vi "cursor window logic V3.vi"(4 "h. offset":dbl, 6 "CursIdx":i32, 7 "cursor window action":T2=enum."check", 8 "window":dbl=nan, 9 "center":dbl=nan, 10 "cursor window in":refnum<vi>, 11 "cursor window init":T1={"left"=2378.60310421286, "right "=2421.6740576496672, "center"=2421.6740576496672, "window"=2421.6740576496672, "cursors"=[], "relative"=0, "absolute"=0, "fixed vertical offset"=2421.6740576496672, "vertical offset"=2421.6740576496672, "skew"=2421.6740576496672, "default window frac"=2421.6740576496672, "kind"=enum."skewed", "skew.left"=2421.6740576496672, "skew.right"=2421.6740576496672, "Plot ref"=refnum, "wing order"=enum."back"}) -> (2 "cursor window out":refnum<vi>, 3 "cursor window out":T1={"left"=2378.60310421286, "right "=2421.6740576496672, "center"=2421.6740576496672, "window"=2421.6740576496672, "cursors"=[], "relative"=0, "absolute"=0, "fixed vertical offset"=2421.6740576496672, "vertical offset"=2421.6740576496672, "skew"=2421.6740576496672, "default window frac"=2421.6740576496672, "kind"=enum."skewed", "skew.left"=2421.6740576496672, "skew.right"=2421.6740576496672, "Plot ref"=refnum, "wing order"=enum."back"})   [LabVIEW 2018]
uses:
  stack action -- control.ctl
  cursor window action.ctl
  cursor winow.ctl
  cursor window state.ctl
  cursor action.ctl
  cursor sate.ctl
  range multiplier action.ctl
  2Dwindow.ctl
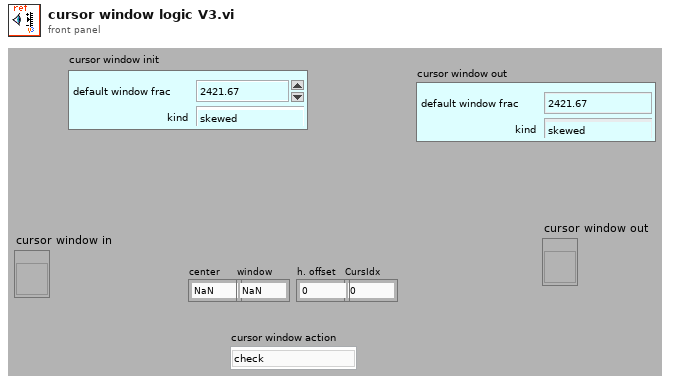
[diagram p1: front panel]
types:
  T1 = typedef "cursor winow.ctl" = cluster{"left":dbl, "right ":dbl, "center":dbl, "window":dbl, "cursors":i32[], "relative":i32, "absolute":i32, "fixed vertical offset":dbl, "vertical offset":dbl, "skew":dbl, "default window frac":dbl, "kind":enum16{"symmetric", "skewed", "fancy"}, "skew.left":dbl, "skew.right":dbl, "Plot ref":refnum<vi>, "wing order":enum16{"forw", "back"}}
  T2 = typedef "cursor window action.ctl" = enum16{"balance", "h. offset change", "cursor moves", "change center", "change window", "init", "check", "reset", "set y to middle", "idle", "-write all Y", "-write left.X", "-write center.X", "-write right.X", "-write all X", "-change center", "-change window", "-change skew", "-read cursor 2", "-read cursor 1", "-read cursor 0", "-read all cursors", "-reset", "-read plot scale", "-set y to middle", "-Q: center.Y is visible", "-Q: window is visible", "-parse center.Y", "-right left from center", "-left move", "-right move", "-set center.Y", "-empty", "-set cursors to default", "-check", "-write center.Y", "-copy cursor 1", "-copy cursor 0", "-copy cursor 2", "move right", "move left", "shrink", "broaden", "skew up", "skew down", "-write plot scale", "zoom X", "change cen&win", "zoom to all data", "color--red", "color--green", "color--yellow", "read", "zoom out", "zoom in", "slide right", "slide left", "set range aspect ratio to 1"}
  T3 = typedef "cursor window state.ctl" = cluster{"right.Y":dbl, "right.X":dbl, "left.X":dbl, "left.Y":dbl, "center.X":dbl, "center.Y":dbl, "scale.x.max":dbl, "scale.x.min":dbl, "scale.y.range":dbl, "scale.y.min":dbl, "scale.x.range":dbl, "scale.y.max":dbl, "skew":dbl, "cursor":i32, "scale.x.center":dbl, "scale.x.halfwidth":dbl, "scale.y.center":dbl, "scale.y.halfwidth":dbl}
  T4 = typedef "stack action -- control.ctl" = enum16{"push", "pop", "check", "init"}
  T5 = cluster{"center":dbl, "window":dbl, "h.offset":dbl, "cursor window":T1}
  T6 = cluster{"right.Y":dbl, "right.X":dbl, "left.X":dbl, "left.Y":dbl, "center.X":dbl, "center.Y":dbl, "scale.x.max":dbl, "scale.x.min":dbl, "scale.y.range":dbl, "scale.y.min":dbl, "scale.x.range":dbl, "scale.y.max":dbl, "skew":dbl, "cursor":i32, "scale.x.center":dbl, "scale.x.halfwidth":dbl, "scale.y.center":dbl, "scale.y.halfwidth":dbl}
  T7 = cluster{"left":dbl, "right ":dbl, "center":dbl, "window":dbl, "cursors":i32[], "relative":i32, "absolute":i32, "fixed vertical offset":dbl, "vertical offset":dbl, "skew":dbl, "default window frac":dbl, "kind":enum16{"symmetric", "skewed", "fancy"}, "skew.left":dbl, "skew.right":dbl, "Plot ref":refnum<vi>, "wing order":enum16{"forw", "back"}}
  T8 = typedef "cursor action.ctl" = enum16{"range", "read", "write", "check", "zoom out", "smart zoom out", "zoom to aspect ratio 1", "zoom to win", "zoom out 20%", "zoom in 20%", "-empty", "smart zoom out&aspect", "move range left 20%", "move range right 20%", "move range up 20%", "move range down 20%", "zoom to X win", "zoom to Y win", "zoom out X", "zoom out Y", "zoom in X", "zoom in Y", "check plot scale"}
  T9 = typedef "2Dwindow.ctl" = cluster{"window y":dbl, "center x":dbl, "center y":dbl, "window x":dbl}
  T10 = typedef "range multiplier action.ctl" = enum16{"shift", "zoom", "check"}
  T11 = typedef "comparison control.ctl" = enum16{"not a number", "above", "in range", "below"}
  T12 = typedef "2Dwindow-bounds.ctl" = cluster{"min y":dbl, "max x":dbl, "min x":dbl, "max y":dbl}
  T13 = typedef "cursor sate.ctl" = enum16{"normal", "alert", "fuzzy", "interesting", "boring", "colored"}
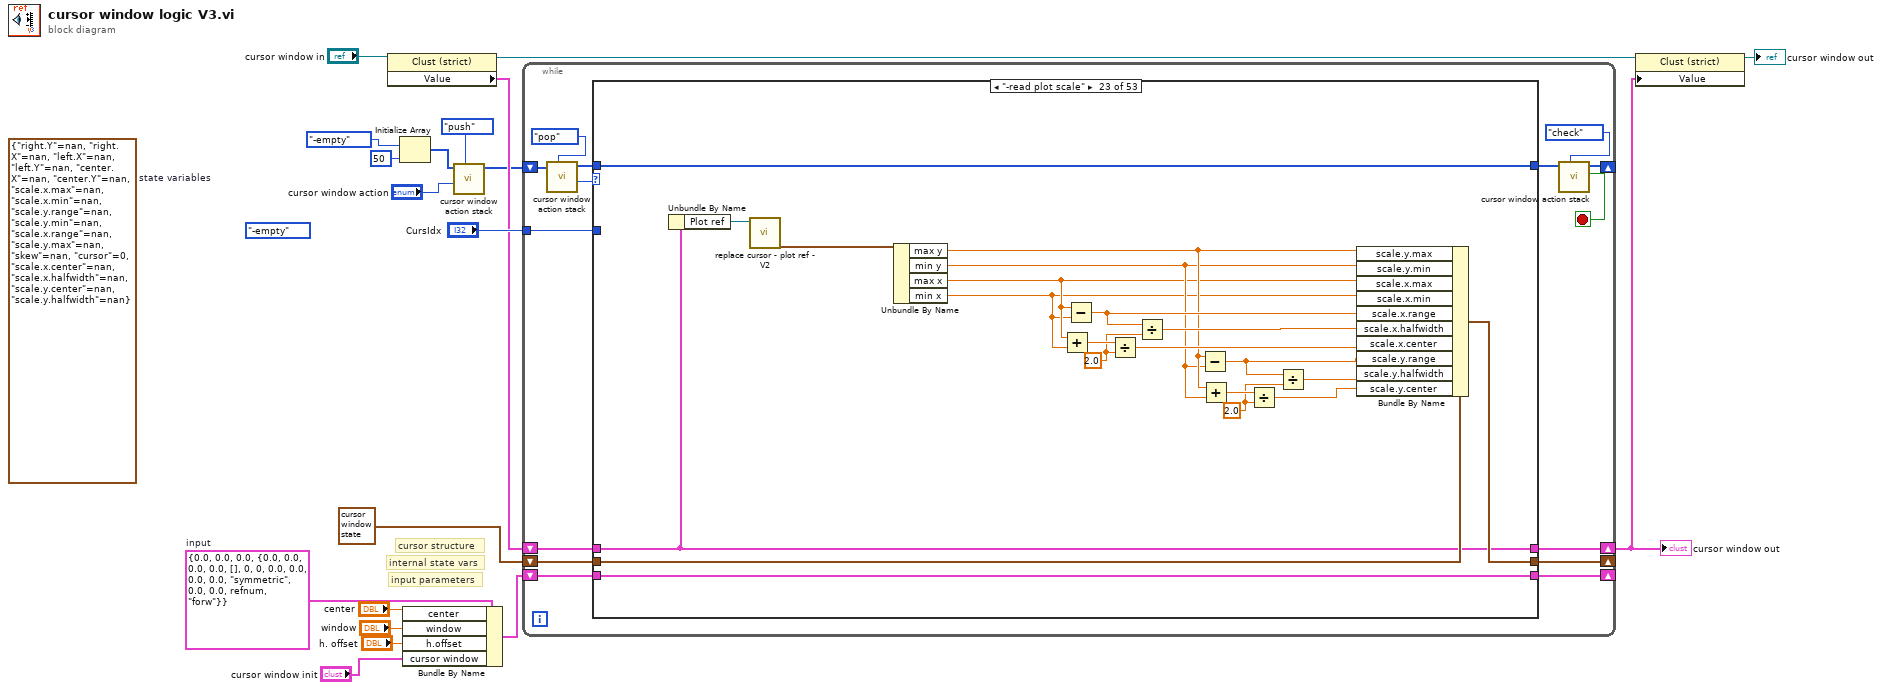
[diagram p0: block diagram]
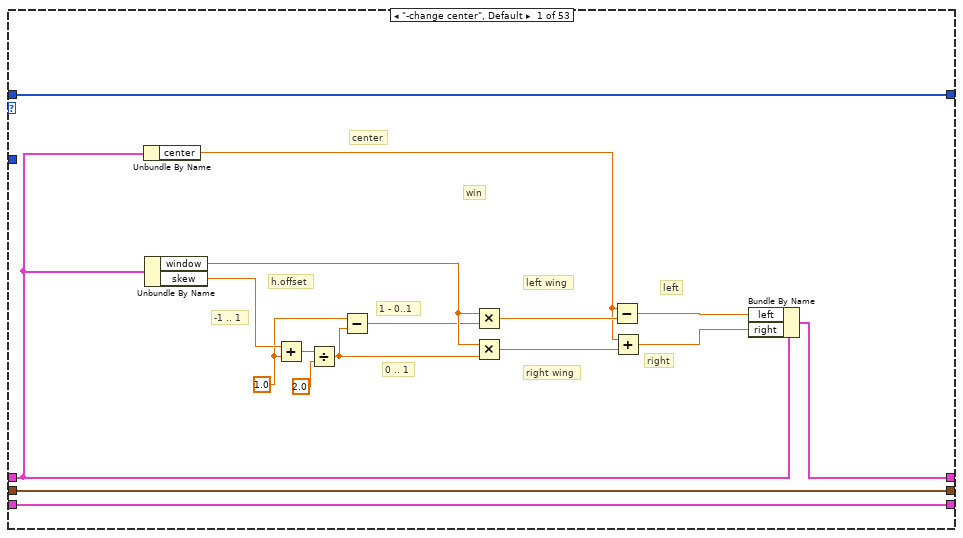
[diagram p2: hidden frame]
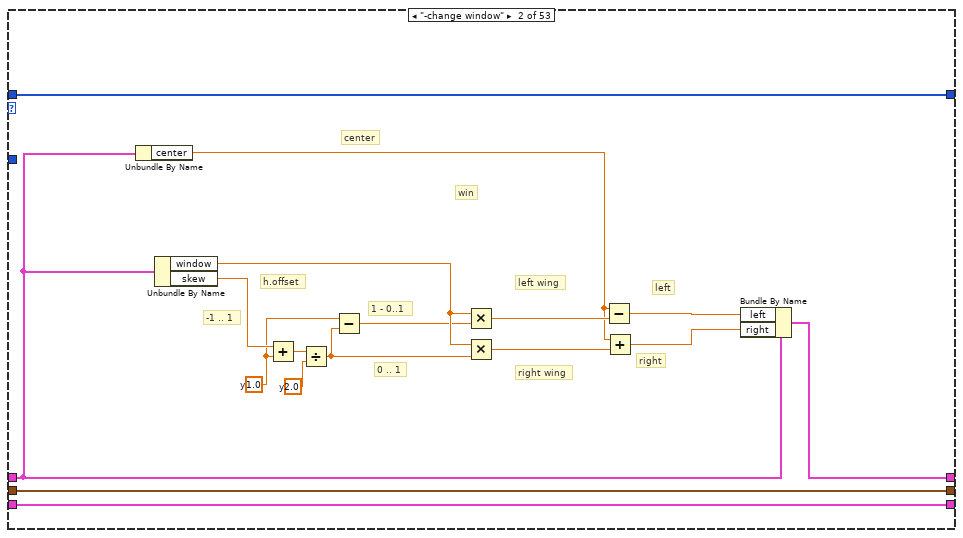
[diagram p3: hidden frame]
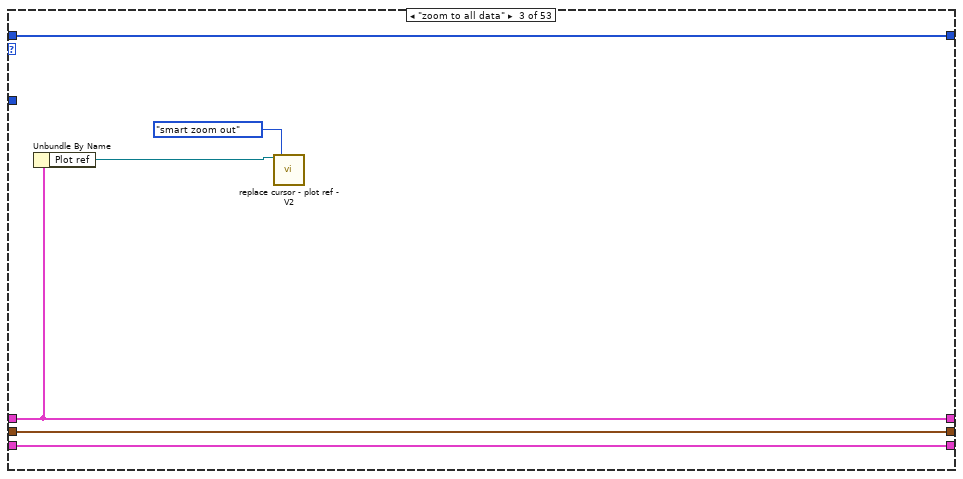
[diagram p4: hidden frame]
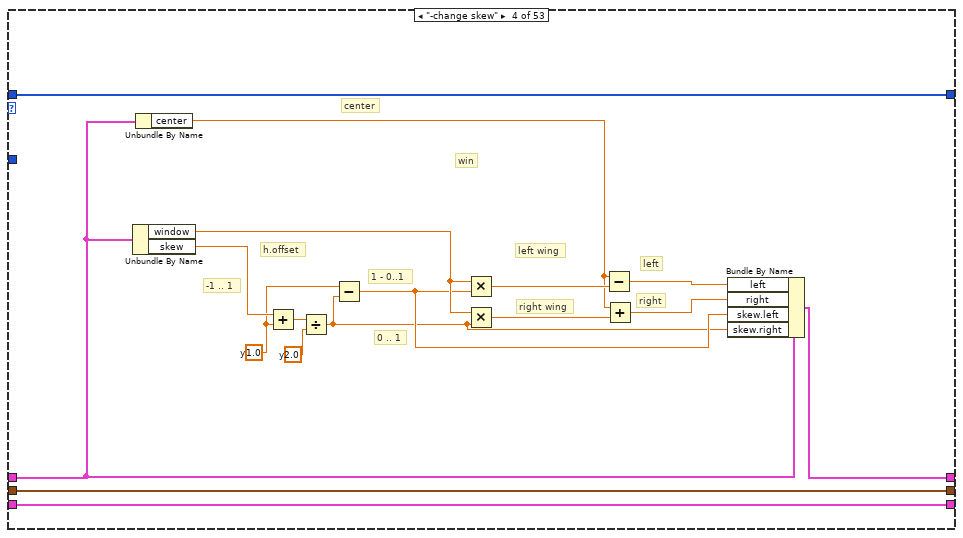
[diagram p5: hidden frame]
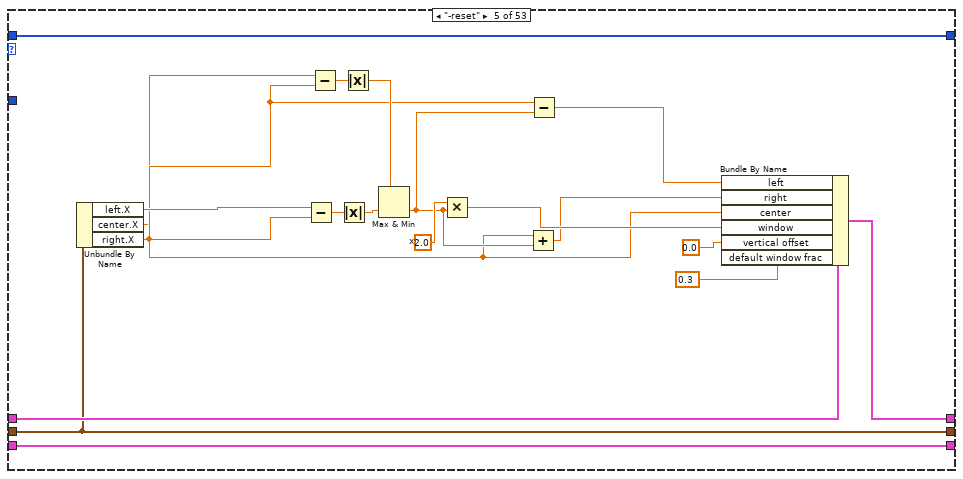
[diagram p6: hidden frame]
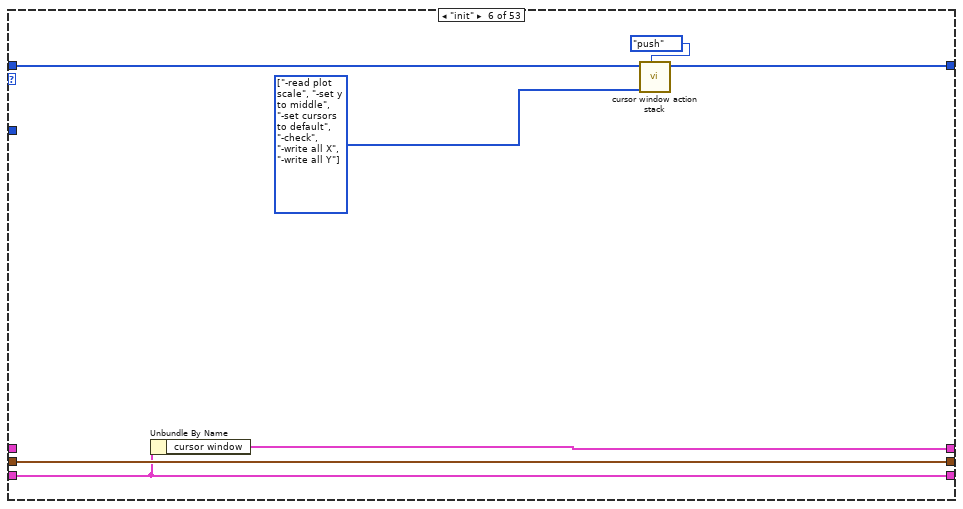
[diagram p7: hidden frame]
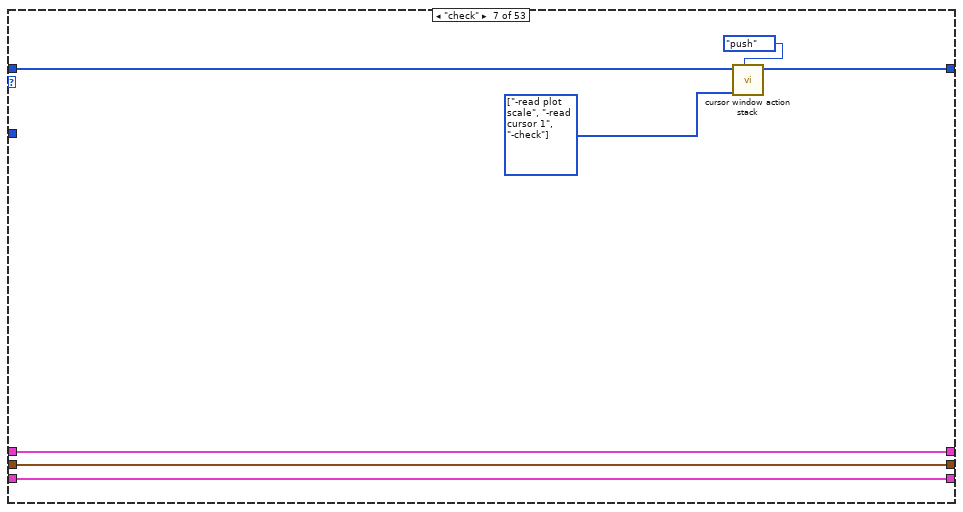
[diagram p8: hidden frame]
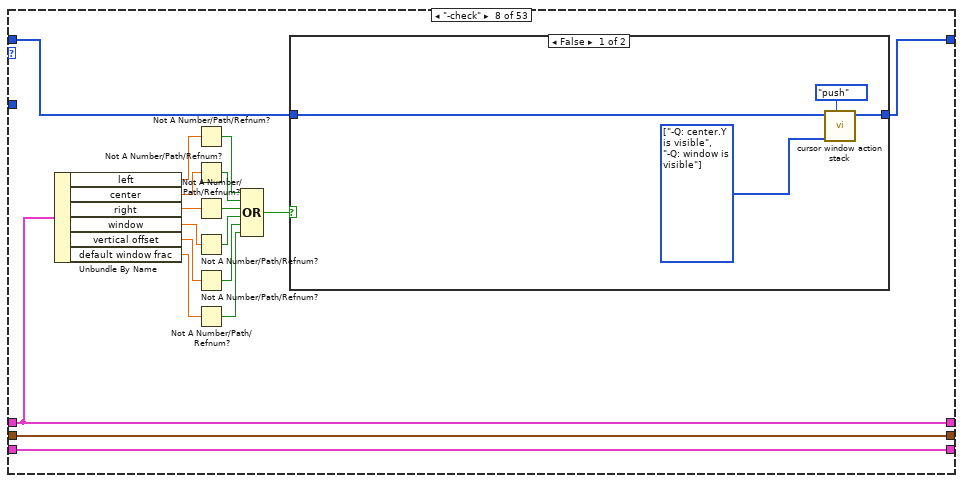
[diagram p9: hidden frame]
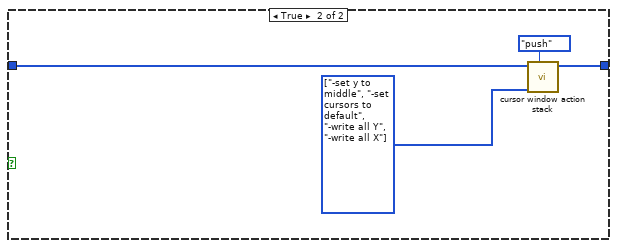
[diagram p10: hidden frame]
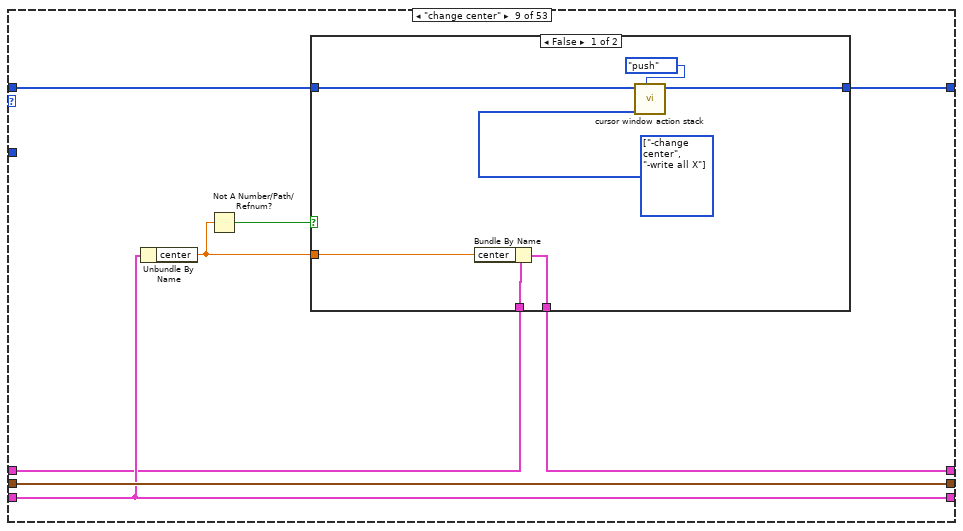
[diagram p11: hidden frame]
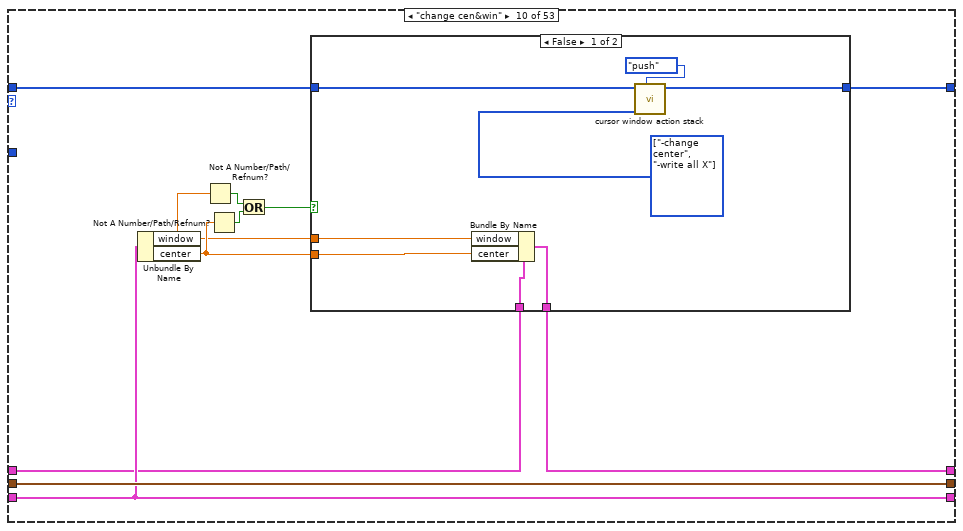
[diagram p13: hidden frame]
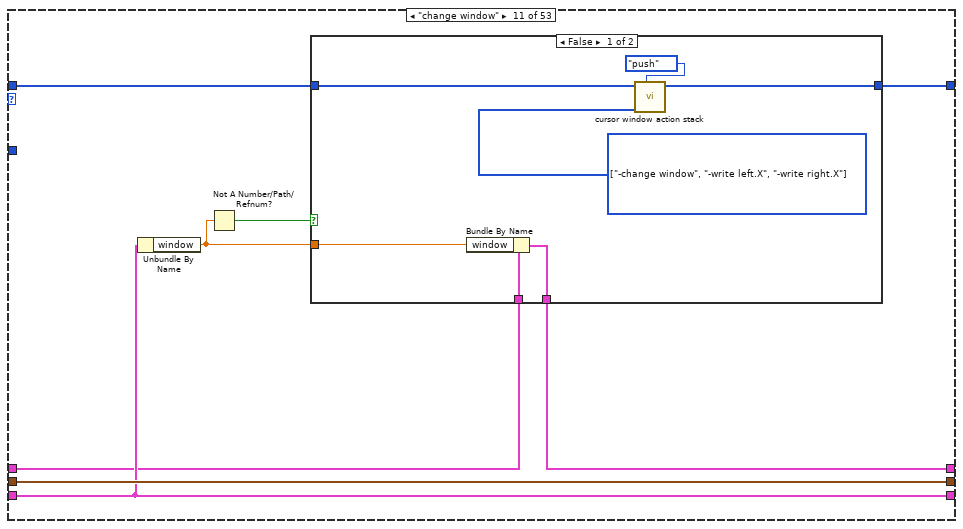
[diagram p15: hidden frame]
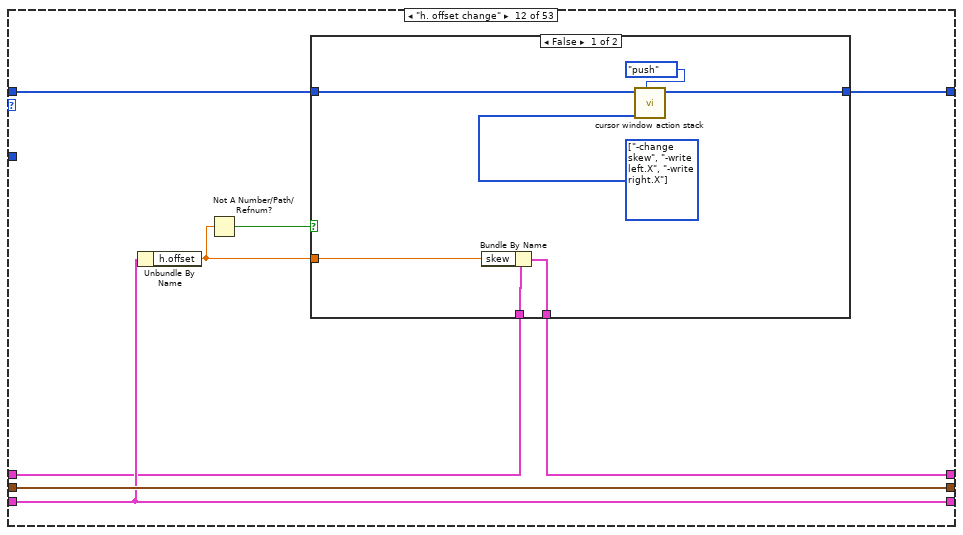
[diagram p17: hidden frame]
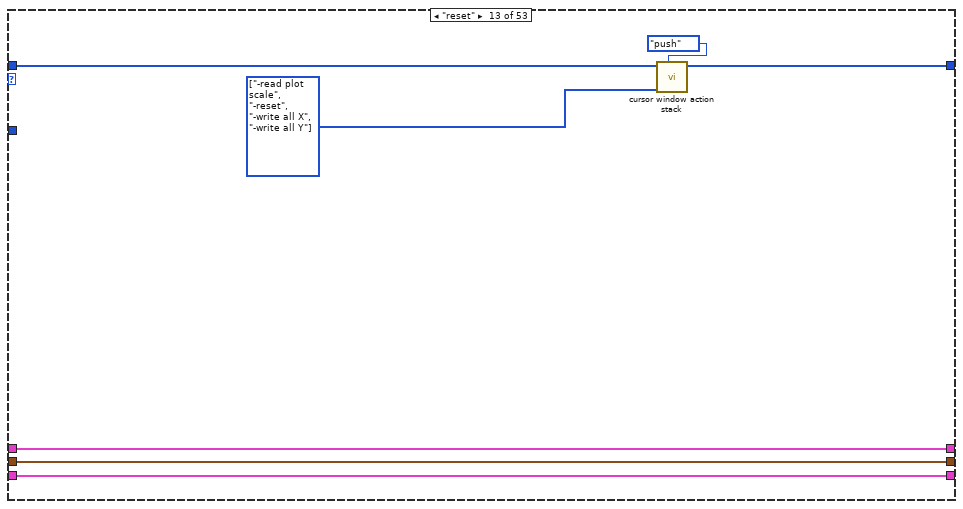
[diagram p19: hidden frame]
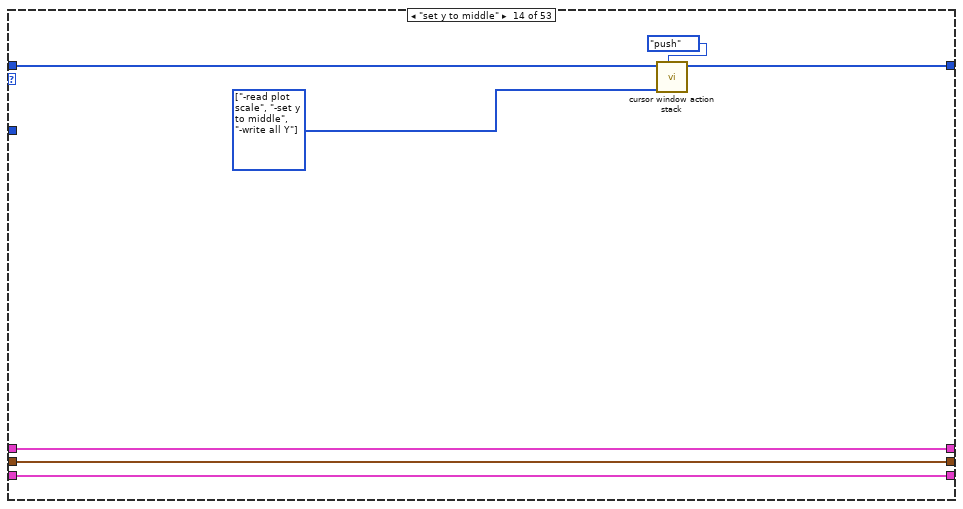
[diagram p20: hidden frame]
diagram:
  (unwired) cursor_window_action."-empty" ("cursor window action")
  w18 = T5 {"center"=0.0, "window"=0.0, "h.offset"=0.0, "cursor window"={"left"=0.0, "right "=0.0, "center"=0.0, "window"=0.0, "cursors"=[], "relative"=0, "absolute"=0, "fixed vertical offset"=0.0, "vertical offset"=0.0, "skew"=0.0, "default window frac"=0.0, "kind"=enum."symmetric", "skew.left"=0.0, "skew.right"=0.0, "Plot ref"=refnum, "wing order"=enum."forw"}}  # input
  (unwired) T6 {"right.Y"=nan, "right.X"=nan, "left.X"=nan, "left.Y"=nan, "center.X"=nan, "center.Y"=nan, "scale.x.max"=nan, "scale.x.min"=nan, "scale.y.range"=nan, "scale.y.min"=nan, "scale.x.range"=nan, "scale.y.max"=nan, "skew"=nan, "cursor"=0, "scale.x.center"=nan, "scale.x.halfwidth"=nan, "scale.y.center"=nan, "scale.y.halfwidth"=nan}  # state variables
  # "input parameters"
  # "internal state vars"
  # "cursor structure"
  n1 = property class="Clust (strict)"(reference="cursor window in") -> (reference out=w19:refnum<vi>, "Value"=w12:T7)  [unwired: 1 in, 1 out]
  n2 = Initialize Array(cursor_window_action."-empty" ("cursor window action"), 50 ("dimension size")) -> (w5:T2[])
  n3 = Bundle By Name(cluster=w18, "center"="center", "window"="window", "h.offset"="h. offset", "cursor window"="cursor window init") -> (w14:T5)
  n4 = call "cursor window action stack.vi"("stack action"=stack_action_--_control."push", "cursor window action"="cursor window action", "command stack"=w5) -> ("command stack out"=w4:T2[])  [unwired: 6 in, 2 out]
  n5 = while {
    shift-right: [w27] -> _
    shift-left: w4 -> [w33]
    shift-right: [w20] -> w11
    shift-left: w12 -> [w34]
    shift-right: [w24] -> _
    shift-left: w14 -> [w25]
    shift-right: [w22] -> _
    shift-left: T3 {"right.Y"=nan, "right.X"=nan, "left.X"=nan, "left.Y"=nan, "center.X"=nan, "center.Y"=nan, "scale.x.max"=nan, "scale.x.min"=nan, "scale.y.range"=nan, "scale.y.min"=nan, "scale.x.range"=nan, "scale.y.max"=nan, "skew"=nan, "cursor"=0, "scale.x.center"=nan, "scale.x.halfwidth"=nan, "scale.y.center"=nan, "scale.y.halfwidth"=nan} ("state variables") -> [w23]
    tunnel: "CursIdx" -> [w21]
    stop <- w26 stop-if-true
    n6 = call "cursor window action stack.vi"("stack action"=stack_action_--_control."pop", "command stack"=w33) -> ("cursor window action out"=w32:T2, "command stack out"=w30:T2[])  [unwired: 7 in, 1 out]
    n7 = case shown="\"-read plot scale\"" w32 {
      tunnel: w34 -> [w36 w53 w71 w78 w100 _ w118 w128 w152 w173 w190 w207 w223 w230 w247 w281 w316 w355 w387 w398 w405 w424 w437 w463 w478 w484 w490 w496 w502 w508 w515 w539 w545 w565 w571 w584 w605 w644 w678 w718 w739 w759 w779 w800 w814 w831 w850 w863 w872 w895 w899 w912 w926]
      tunnel: [w40 w57 w74 w82 w99 w112 w121 w125 w157 w177 w195 w212 w226 w233 w244 w278 w318 w356 w388 w396 w414 w430 w448 w464 w479 w485 w491 w497 w503 w509 w513 w540 w553 w566 w580 w588 w609 w642 w680 w735 w755 w775 w795 w813 w828 w845 w859 w871 w893 w897 w911 w925 w939] -> w28
      tunnel: w30 -> [w40 w57 w74 w82 w99 w113 w122 w126 w156 w176 w194 w211 w227 w234 w244 w278 w318 w343 w388 w396 w414 w430 w448 w464 w479 w485 w491 w497 w503 w509 w514 w541 w554 w567 w581 w589 w610 w642 w681 w735 w755 w775 w795 w813 w828 w845 w859 w871 w893 w897 w911 w925 w939]
      tunnel: w25 -> [w37 w54 w72 w79 w98 w116 w119 w129 w155 w175 w193 w210 w229 w236 w246 w280 w317 w348 w385 w399 w413 w429 w451 w465 w480 w486 w492 w498 w504 w510 w521 w535 w551 w561 w578 w585 w606 w660 w685 w720 w741 w761 w781 w802 w820 w838 w852 w865 w874 w896 w901 w915 w929]
      tunnel: [w37 w54 w72 w79 w98 w116 w119 w129 w155 w175 w193 w210 w229 w236 w246 w280 w317 w348 w385 w399 w413 w429 w451 w465 w480 w486 w492 w498 w504 w510 w521 w535 w551 w561 w578 w585 w606 w660 w685 w720 w741 w761 w781 w802 w820 w838 w852 w865 w874 w896 w901 w915 w929] -> w24
      tunnel: w23 -> [w39 w56 w73 w81 w97 w117 w120 w130 w158 w178 w196 w213 w228 w235 w245 w279 w322 w349 w386 w401 w410 w428 w450 w462 w477 w483 w489 w495 w501 w507 w517 w536 w552 w562 w579 w586 w607 w648 w684 w721 w742 w762 w782 w799 w821 w839 w853 w862 w882 w894 w905 w919 w933]
      tunnel: [w39 w56 w73 w81 w97 w117 w120 w130 w158 w178 w196 w213 w228 w235 w245 w279 w321 w349 w386 w401 w409 w428 w449 w462 w477 w483 w489 w495 w501 w507 w516 w536 w552 w562 w579 w586 w607 w651 w684 w721 w742 w762 w782 w799 w821 w839 w853 w862 w881 w894 w904 w918 w932] -> w22
      tunnel: w21 -> [_ _ _ _ _ _ _ _ _ _ _ _ _ _ _ _ _ w346 _ _ _ _ _ _ _ _ _ _ _ _ _ _ _ _ _ _ _ _ _ _ _ _ _ _ _ _ _ _ _ _ _ _ _]
      tunnel: [w35 w52 w71 w77 w93 w111 w118 w128 w151 w172 w189 w206 w223 w230 w237 w271 w316 w347 w387 w397 w404 w420 w437 w463 w478 w484 w490 w496 w502 w508 w515 w538 w544 w564 w570 w587 w608 w640 w677 w718 w739 w759 w779 w800 w814 w831 w850 w863 w872 w895 w899 w912 w926] -> w20
      frame "-change center", Default {
        w45 = 1.0 ("y")
        # "1 - 0..1"
        # "right"
        # "left"
        # "win"
        # "h.offset"
        # "center"
        # "left wing"
        # "right wing"
        # "0 .. 1"
        # "-1 .. 1"
        n8 = Unbundle By Name(w36) -> ("center"=w38:dbl)
        n9 = Unbundle By Name(w36) -> ("window"=w50:dbl, "skew"=w51:dbl)
        n10 = Add(x=w51, y=w45) -> (x+y=w46:dbl)
        n11 = Divide(x=w46, y=2.0) -> (x/y=w42:dbl)
        n12 = Subtract(x=w45, y=w42) -> (x-y=w41:dbl)
        n13 = Multiply(x=w50, y=w41) -> (x*y=w44:dbl)
        n14 = Multiply(x=w50, y=w42) -> (x*y=w43:dbl)
        n15 = Subtract(x=w38, y=w44) -> (x-y=w49:dbl)
        n16 = Add(x=w38, y=w43) -> (x+y=w48:dbl)
        n17 = Bundle By Name(cluster=w36, "left"=w49, "right"=w48) -> (w35:T1)
      }
      frame "-change window" {
        w62 = 1.0  # y
        w64 = 2.0  # y
        # "1 - 0..1"
        # "right"
        # "left"
        # "win"
        # "h.offset"
        # "center"
        # "left wing"
        # "right wing"
        # "0 .. 1"
        # "-1 .. 1"
        n18 = Unbundle By Name(w53) -> ("center"=w55:dbl)
        n19 = Unbundle By Name(w53) -> ("window"=w67:dbl, "skew"=w68:dbl)
        n20 = Add(x=w68, y=w62) -> (x+y=w63:dbl)
        n21 = Divide(x=w63, y=w64) -> (x/y=w59:dbl)
        n22 = Subtract(x=w62, y=w59) -> (x-y=w58:dbl)
        n23 = Multiply(x=w67, y=w58) -> (x*y=w61:dbl)
        n24 = Multiply(x=w67, y=w59) -> (x*y=w60:dbl)
        n25 = Subtract(x=w55, y=w61) -> (x-y=w66:dbl)
        n26 = Add(x=w55, y=w60) -> (x+y=w65:dbl)
        n27 = Bundle By Name(cluster=w53, "left"=w66, "right"=w65) -> (w52:T1)
      }
      frame "zoom to all data" {
        n28 = Unbundle By Name(w71) -> ("Plot ref"=w70:refnum<vi>)
        n29 = call "replace cursor - plot ref - V2.vi"("Plot ref in"=w70, "cursor action"=cursor_action."smart zoom out") -> ()  [unwired: 14 in, 4 out]
      }
      frame "-change skew" {
        w85 = 1.0  # y
        w87 = 2.0  # y
        # "1 - 0..1"
        # "right"
        # "left"
        # "win"
        # "h.offset"
        # "center"
        # "left wing"
        # "right wing"
        # "0 .. 1"
        # "-1 .. 1"
        n30 = Unbundle By Name(w78) -> ("window"=w90:dbl, "skew"=w91:dbl)
        n31 = Unbundle By Name(w78) -> ("center"=w80:dbl)
        n32 = Add(x=w91, y=w85) -> (x+y=w86:dbl)
        n33 = Divide(x=w86, y=w87) -> (x/y=w75:dbl)
        n34 = Subtract(x=w85, y=w75) -> (x-y=w76:dbl)
        n35 = Multiply(x=w90, y=w76) -> (x*y=w84:dbl)
        n36 = Multiply(x=w90, y=w75) -> (x*y=w83:dbl)
        n37 = Subtract(x=w80, y=w84) -> (x-y=w89:dbl)
        n38 = Add(x=w80, y=w83) -> (x+y=w88:dbl)
        n39 = Bundle By Name(cluster=w78, "left"=w89, "right"=w88, "skew.left"=w76, "skew.right"=w75) -> (w77:T1)
      }
      frame "-reset" {
        w106 = 2.0  # x
        n40 = Unbundle By Name(w97) -> ("left.X"=w96:dbl, "center.X"=w94:dbl, "right.X"=w95:dbl)
        n41 = Subtract(x=w96, y=w95) -> (x-y=w109:dbl)
        n42 = Subtract(x=w94, y=w95) -> (x-y=w110:dbl)
        n43 = Absolute Value(x=w109) -> (abs(x)=w107:dbl)
        n44 = Absolute Value(x=w110) -> (abs(x)=w108:dbl)
        n45 = Max & Min(x=w108, y=w107) -> (min(x,y)=w104:dbl)  [unwired: 1 out]
        n46 = Multiply(x=w106, y=w104) -> (x*y=w105:dbl)
        n47 = Add(x=w95, y=w104) -> (x+y=w102:dbl)
        n48 = Subtract(x=w95, y=w104) -> (x-y=w103:dbl)
        n49 = Bundle By Name(cluster=w100, "left"=w103, "right"=w102, "center"=w95, "window"=w105, "vertical offset"=0.0, "default window frac"=0.3) -> (w93:T1)
      }
      frame "init" {
        w114 = T2[] [enum."-read plot scale", enum."-set y to middle", enum."-set cursors to default", enum."-check", enum."-write all X", enum."-write all Y"] items=["balance", "h. offset change", "cursor moves", "change center", "change window", "init", "check", "reset", "set y to middle", "idle", "-write all Y", "-write left.X", "-write center.X", "-write right.X", "-write all X", "-change center", "-change window", "-change skew", "-read cursor 2", "-read cursor 1", "-read cursor 0", "-read all cursors", "-reset", "-read plot scale", "-set y to middle", "-Q: center.Y is visible", "-Q: window is visible", "-parse center.Y", "-right left from center", "-left move", "-right move", "-set center.Y", "-empty", "-set cursors to default", "-check", "-write center.Y", "-copy cursor 1", "-copy cursor 0", "-copy cursor 2", "move right", "move left", "shrink", "broaden", "skew up", "skew down", "-write plot scale", "zoom X", "change cen&win", "zoom to all data", "color--red", "color--green", "color--yellow", "read", "zoom out", "zoom in", "slide right", "slide left", "set range aspect ratio to 1"]
        n50 = Unbundle By Name(w116) -> ("cursor window"=w111:T1)
        n51 = call "cursor window action stack.vi"("stack action"=stack_action_--_control."push", "action list"=w114, "command stack"=w113) -> ("command stack out"=w112:T2[])  [unwired: 6 in, 2 out]
      }
      frame "check" {
        w123 = T2[] [enum."-read plot scale", enum."-read cursor 1", enum."-check"] items=["balance", "h. offset change", "cursor moves", "change center", "change window", "init", "check", "reset", "set y to middle", "idle", "-write all Y", "-write left.X", "-write center.X", "-write right.X", "-write all X", "-change center", "-change window", "-change skew", "-read cursor 2", "-read cursor 1", "-read cursor 0", "-read all cursors", "-reset", "-read plot scale", "-set y to middle", "-Q: center.Y is visible", "-Q: window is visible", "-parse center.Y", "-right left from center", "-left move", "-right move", "-set center.Y", "-empty", "-set cursors to default", "-check", "-write center.Y", "-copy cursor 1", "-copy cursor 0", "-copy cursor 2", "move right", "move left", "shrink", "broaden", "skew up", "skew down", "-write plot scale", "zoom X", "change cen&win", "zoom to all data", "color--red", "color--green", "color--yellow", "read", "zoom out", "zoom in", "slide right", "slide left", "set range aspect ratio to 1"]
        n52 = call "cursor window action stack.vi"("stack action"=stack_action_--_control."push", "action list"=w123, "command stack"=w122) -> ("command stack out"=w121:T2[])  [unwired: 6 in, 2 out]
      }
      frame "-check" {
        n53 = Unbundle By Name(w128) -> ("left"=w140:dbl, "center"=w139:dbl, "right"=w141:dbl, "window"=w142:dbl, "vertical offset"=w134:dbl, "default window frac"=w133:dbl)
        n54 = Not A Number/Path/Refnum?(number/path/refnum=w140) -> (NaN/Path/Refnum?=w138:bool)
        n55 = Not A Number/Path/Refnum?(number/path/refnum=w139) -> (NaN/Path/Refnum?=w137:bool)
        n56 = Not A Number/Path/Refnum?(number/path/refnum=w141) -> (NaN/Path/Refnum?=w136:bool)
        n57 = Not A Number/Path/Refnum?(number/path/refnum=w142) -> (NaN/Path/Refnum?=w135:bool)
        n58 = Not A Number/Path/Refnum?(number/path/refnum=w134) -> (NaN/Path/Refnum?=w131:bool)
        n59 = Not A Number/Path/Refnum?(number/path/refnum=w133) -> (NaN/Path/Refnum?=w132:bool)
        n60 = Compound Arithmetic op=OR(w138, w137, w136, w135, w131, w132) -> (w127:bool)
        n61 = case shown="False" w127 {
          tunnel: w126 -> [w144 w148]
          tunnel: [w143 w147] -> w125
          frame False {
            w145 = T2[] [enum."-Q: center.Y is visible", enum."-Q: window is visible"] items=["balance", "h. offset change", "cursor moves", "change center", "change window", "init", "check", "reset", "set y to middle", "idle", "-write all Y", "-write left.X", "-write center.X", "-write right.X", "-write all X", "-change center", "-change window", "-change skew", "-read cursor 2", "-read cursor 1", "-read cursor 0", "-read all cursors", "-reset", "-read plot scale", "-set y to middle", "-Q: center.Y is visible", "-Q: window is visible", "-parse center.Y", "-right left from center", "-left move", "-right move", "-set center.Y", "-empty", "-set cursors to default", "-check", "-write center.Y", "-copy cursor 1", "-copy cursor 0", "-copy cursor 2", "move right", "move left", "shrink", "broaden", "skew up", "skew down", "-write plot scale", "zoom X", "change cen&win", "zoom to all data", "color--red", "color--green", "color--yellow", "read", "zoom out", "zoom in", "slide right", "slide left", "set range aspect ratio to 1"]
            n62 = call "cursor window action stack.vi"("stack action"=stack_action_--_control."push", "action list"=w145, "command stack"=w144) -> ("command stack out"=w143:T2[])  [unwired: 6 in, 2 out]
          }
          frame True {
            w149 = T2[] [enum."-set y to middle", enum."-set cursors to default", enum."-write all Y", enum."-write all X"] items=["balance", "h. offset change", "cursor moves", "change center", "change window", "init", "check", "reset", "set y to middle", "idle", "-write all Y", "-write left.X", "-write center.X", "-write right.X", "-write all X", "-change center", "-change window", "-change skew", "-read cursor 2", "-read cursor 1", "-read cursor 0", "-read all cursors", "-reset", "-read plot scale", "-set y to middle", "-Q: center.Y is visible", "-Q: window is visible", "-parse center.Y", "-right left from center", "-left move", "-right move", "-set center.Y", "-empty", "-set cursors to default", "-check", "-write center.Y", "-copy cursor 1", "-copy cursor 0", "-copy cursor 2", "move right", "move left", "shrink", "broaden", "skew up", "skew down", "-write plot scale", "zoom X", "change cen&win", "zoom to all data", "color--red", "color--green", "color--yellow", "read", "zoom out", "zoom in", "slide right", "slide left", "set range aspect ratio to 1"]
            n63 = call "cursor window action stack.vi"("stack action"=stack_action_--_control."push", "action list"=w149, "command stack"=w148) -> ("command stack out"=w147:T2[])  [unwired: 6 in, 2 out]
          }
        }
      }
      frame "change center" {
        n64 = Unbundle By Name(w155) -> ("center"=w153:dbl)
        n65 = Not A Number/Path/Refnum?(number/path/refnum=w153) -> (NaN/Path/Refnum?=w154:bool)
        n66 = case shown="False" w154 {
          tunnel: [w165 w166] -> w157
          tunnel: w156 -> [w164 w166]
          tunnel: w152 -> [w161 w167]
          tunnel: w153 -> [w160 _]
          tunnel: [w159 w167] -> w151
          frame False {
            w162 = T2[] [enum."-change center", enum."-write all X"] items=["balance", "h. offset change", "cursor moves", "change center", "change window", "init", "check", "reset", "set y to middle", "idle", "-write all Y", "-write left.X", "-write center.X", "-write right.X", "-write all X", "-change center", "-change window", "-change skew", "-read cursor 2", "-read cursor 1", "-read cursor 0", "-read all cursors", "-reset", "-read plot scale", "-set y to middle", "-Q: center.Y is visible", "-Q: window is visible", "-parse center.Y", "-right left from center", "-left move", "-right move", "-set center.Y", "-empty", "-set cursors to default", "-check", "-write center.Y", "-copy cursor 1", "-copy cursor 0", "-copy cursor 2", "move right", "move left", "shrink", "broaden", "skew up", "skew down", "-write plot scale", "zoom X", "change cen&win", "zoom to all data", "color--red", "color--green", "color--yellow", "read", "zoom out", "zoom in", "slide right", "slide left", "set range aspect ratio to 1"]
            n67 = Bundle By Name(cluster=w161, "center"=w160) -> (w159:T1)
            n68 = call "cursor window action stack.vi"("stack action"=stack_action_--_control."push", "action list"=w162, "command stack"=w164) -> ("command stack out"=w165:T2[])  [unwired: 6 in, 2 out]
          }
          frame True {
          }
        }
      }
      frame "change cen&win" {
        n69 = Unbundle By Name(w175) -> ("window"=w168:dbl, "center"=w174:dbl)
        n70 = Not A Number/Path/Refnum?(number/path/refnum=w168) -> (NaN/Path/Refnum?=w171:bool)
        n71 = Not A Number/Path/Refnum?(number/path/refnum=w174) -> (NaN/Path/Refnum?=w170:bool)
        n72 = Or(x=w171, y=w170) -> (x .or. y?=w169:bool)
        n73 = case shown="False" w169 {
          tunnel: [w186 w187] -> w177
          tunnel: w176 -> [w185 w187]
          tunnel: w173 -> [w182 w188]
          tunnel: w174 -> [w181 _]
          tunnel: [w180 w188] -> w172
          tunnel: w168 -> [w179 _]
          frame False {
            w183 = T2[] [enum."-change center", enum."-write all X"] items=["balance", "h. offset change", "cursor moves", "change center", "change window", "init", "check", "reset", "set y to middle", "idle", "-write all Y", "-write left.X", "-write center.X", "-write right.X", "-write all X", "-change center", "-change window", "-change skew", "-read cursor 2", "-read cursor 1", "-read cursor 0", "-read all cursors", "-reset", "-read plot scale", "-set y to middle", "-Q: center.Y is visible", "-Q: window is visible", "-parse center.Y", "-right left from center", "-left move", "-right move", "-set center.Y", "-empty", "-set cursors to default", "-check", "-write center.Y", "-copy cursor 1", "-copy cursor 0", "-copy cursor 2", "move right", "move left", "shrink", "broaden", "skew up", "skew down", "-write plot scale", "zoom X", "change cen&win", "zoom to all data", "color--red", "color--green", "color--yellow", "read", "zoom out", "zoom in", "slide right", "slide left", "set range aspect ratio to 1"]
            n74 = Bundle By Name(cluster=w182, "window"=w179, "center"=w181) -> (w180:T1)
            n75 = call "cursor window action stack.vi"("stack action"=stack_action_--_control."push", "action list"=w183, "command stack"=w185) -> ("command stack out"=w186:T2[])  [unwired: 6 in, 2 out]
          }
          frame True {
          }
        }
      }
      frame "change window" {
        n76 = Unbundle By Name(w193) -> ("window"=w191:dbl)
        n77 = Not A Number/Path/Refnum?(number/path/refnum=w191) -> (NaN/Path/Refnum?=w192:bool)
        n78 = case shown="False" w192 {
          tunnel: [w203 w204] -> w195
          tunnel: w194 -> [w202 w204]
          tunnel: w190 -> [w199 w205]
          tunnel: w191 -> [w198 _]
          tunnel: [w197 w205] -> w189
          frame False {
            w200 = T2[] [enum."-change window", enum."-write left.X", enum."-write right.X"] items=["balance", "h. offset change", "cursor moves", "change center", "change window", "init", "check", "reset", "set y to middle", "idle", "-write all Y", "-write left.X", "-write center.X", "-write right.X", "-write all X", "-change center", "-change window", "-change skew", "-read cursor 2", "-read cursor 1", "-read cursor 0", "-read all cursors", "-reset", "-read plot scale", "-set y to middle", "-Q: center.Y is visible", "-Q: window is visible", "-parse center.Y", "-right left from center", "-left move", "-right move", "-set center.Y", "-empty", "-set cursors to default", "-check", "-write center.Y", "-copy cursor 1", "-copy cursor 0", "-copy cursor 2", "move right", "move left", "shrink", "broaden", "skew up", "skew down", "-write plot scale", "zoom X", "change cen&win", "zoom to all data", "color--red", "color--green", "color--yellow", "read", "zoom out", "zoom in", "slide right", "slide left", "set range aspect ratio to 1"]
            n79 = Bundle By Name(cluster=w199, "window"=w198) -> (w197:T1)
            n80 = call "cursor window action stack.vi"("stack action"=stack_action_--_control."push", "action list"=w200, "command stack"=w202) -> ("command stack out"=w203:T2[])  [unwired: 6 in, 2 out]
          }
          frame True {
          }
        }
      }
      frame "h. offset change" {
        n81 = Unbundle By Name(w210) -> ("h.offset"=w208:dbl)
        n82 = Not A Number/Path/Refnum?(number/path/refnum=w208) -> (NaN/Path/Refnum?=w209:bool)
        n83 = case shown="False" w209 {
          tunnel: [w220 w221] -> w212
          tunnel: w211 -> [w219 w221]
          tunnel: w207 -> [w216 w222]
          tunnel: w208 -> [w215 _]
          tunnel: [w214 w222] -> w206
          frame False {
            w217 = T2[] [enum."-change skew", enum."-write left.X", enum."-write right.X"] items=["balance", "h. offset change", "cursor moves", "change center", "change window", "init", "check", "reset", "set y to middle", "idle", "-write all Y", "-write left.X", "-write center.X", "-write right.X", "-write all X", "-change center", "-change window", "-change skew", "-read cursor 2", "-read cursor 1", "-read cursor 0", "-read all cursors", "-reset", "-read plot scale", "-set y to middle", "-Q: center.Y is visible", "-Q: window is visible", "-parse center.Y", "-right left from center", "-left move", "-right move", "-set center.Y", "-empty", "-set cursors to default", "-check", "-write center.Y", "-copy cursor 1", "-copy cursor 0", "-copy cursor 2", "move right", "move left", "shrink", "broaden", "skew up", "skew down", "-write plot scale", "zoom X", "change cen&win", "zoom to all data", "color--red", "color--green", "color--yellow", "read", "zoom out", "zoom in", "slide right", "slide left", "set range aspect ratio to 1"]
            n84 = Bundle By Name(cluster=w216, "skew"=w215) -> (w214:T1)
            n85 = call "cursor window action stack.vi"("stack action"=stack_action_--_control."push", "action list"=w217, "command stack"=w219) -> ("command stack out"=w220:T2[])  [unwired: 6 in, 2 out]
          }
          frame True {
          }
        }
      }
      frame "reset" {
        w224 = T2[] [enum."-read plot scale", enum."-reset", enum."-write all X", enum."-write all Y"] items=["balance", "h. offset change", "cursor moves", "change center", "change window", "init", "check", "reset", "set y to middle", "idle", "-write all Y", "-write left.X", "-write center.X", "-write right.X", "-write all X", "-change center", "-change window", "-change skew", "-read cursor 2", "-read cursor 1", "-read cursor 0", "-read all cursors", "-reset", "-read plot scale", "-set y to middle", "-Q: center.Y is visible", "-Q: window is visible", "-parse center.Y", "-right left from center", "-left move", "-right move", "-set center.Y", "-empty", "-set cursors to default", "-check", "-write center.Y", "-copy cursor 1", "-copy cursor 0", "-copy cursor 2", "move right", "move left", "shrink", "broaden", "skew up", "skew down", "-write plot scale", "zoom X", "change cen&win", "zoom to all data", "color--red", "color--green", "color--yellow", "read", "zoom out", "zoom in", "slide right", "slide left", "set range aspect ratio to 1"]
        n86 = call "cursor window action stack.vi"("stack action"=stack_action_--_control."push", "action list"=w224, "command stack"=w227) -> ("command stack out"=w226:T2[])  [unwired: 6 in, 2 out]
      }
      frame "set y to middle" {
        w231 = T2[] [enum."-read plot scale", enum."-set y to middle", enum."-write all Y"] items=["balance", "h. offset change", "cursor moves", "change center", "change window", "init", "check", "reset", "set y to middle", "idle", "-write all Y", "-write left.X", "-write center.X", "-write right.X", "-write all X", "-change center", "-change window", "-change skew", "-read cursor 2", "-read cursor 1", "-read cursor 0", "-read all cursors", "-reset", "-read plot scale", "-set y to middle", "-Q: center.Y is visible", "-Q: window is visible", "-parse center.Y", "-right left from center", "-left move", "-right move", "-set center.Y", "-empty", "-set cursors to default", "-check", "-write center.Y", "-copy cursor 1", "-copy cursor 0", "-copy cursor 2", "move right", "move left", "shrink", "broaden", "skew up", "skew down", "-write plot scale", "zoom X", "change cen&win", "zoom to all data", "color--red", "color--green", "color--yellow", "read", "zoom out", "zoom in", "slide right", "slide left", "set range aspect ratio to 1"]
        n87 = call "cursor window action stack.vi"("stack action"=stack_action_--_control."push", "action list"=w231, "command stack"=w234) -> ("command stack out"=w233:T2[])  [unwired: 6 in, 2 out]
      }
      frame "-left move" {
        n88 = Unbundle By Name(w247) -> ("center"=w240:dbl, "skew.left"=w243:dbl, "skew.right"=w242:dbl)
        n89 = Unbundle By Name(w245) -> ("left.X"=w241:dbl)
        n90 = call "Q -- check range -- i -- real.vi"("upper"=w240, "number"=w241) -> ("selector"=w239:T11)  [unwired: 7 in, 2 out]
        n91 = case shown="\"in range\", Default" w239 {
          tunnel: w241 -> [w252 w270]
          tunnel: w242 -> [w258 w269]
          tunnel: [w259 w268] -> w248
          tunnel: [w254 w263] -> w250
          tunnel: w243 -> [w260 w267]
          tunnel: [w256 w262] -> w249
          tunnel: w240 -> [w253 w266]
          tunnel: [enum16{"forw", "back"}."forw" ("wing order") enum16{"forw", "back"}."back" ("wing order")] -> w238
          frame "in range", Default {
            # "right wing"
            # "left wing"
            n92 = Subtract(x=w253, y=w252) -> (x-y=w257:dbl)
            n93 = Divide(x=w257, y=w260) -> (x/y=w259:dbl)
            n94 = Multiply(x=w259, y=w258) -> (x*y=w255:dbl)
            n95 = Subtract(x=w253, y=w257) -> (x-y=w256:dbl)
            n96 = Add(x=w255, y=w253) -> (x+y=w254:dbl)
          }
          frame "above" {
            # "right wing"
            # "left wing"
            n97 = Subtract(x=w270, y=w266) -> (x-y=w265:dbl)
            n98 = Divide(x=w265, y=w269) -> (x/y=w268:dbl)
            n99 = Multiply(x=w268, y=w267) -> (x*y=w264:dbl)
            n100 = Subtract(x=w266, y=w264) -> (x-y=w262:dbl)
            n101 = Add(x=w265, y=w266) -> (x+y=w263:dbl)
          }
        }
        n102 = Bundle By Name(cluster=w247, "left"=w249, "right"=w250, "window"=w248, "wing order"=w238) -> (w237:T1)
      }
      frame "-right move" {
        n103 = Unbundle By Name(w281) -> ("center"=w272:dbl, "skew.left"=w277:dbl, "skew.right"=w276:dbl)
        n104 = Unbundle By Name(w279) -> ("right.X"=w275:dbl)
        n105 = call "Q -- check range -- i -- real.vi"("lower"=w272, "number"=w275) -> ("selector"=w274:T11)  [unwired: 7 in, 2 out]
        n106 = case shown="\"below\"" w274 {
          tunnel: w275 -> [w294 w296]
          tunnel: w276 -> [w293 w302]
          tunnel: [w292 w303] -> w282
          tunnel: [w287 w298] -> w284
          tunnel: w277 -> [w291 w304]
          tunnel: [w286 w300] -> w283
          tunnel: w272 -> [w290 w297]
          tunnel: [enum16{"forw", "back"}."forw" ("wing order") enum16{"forw", "back"}."back" ("wing order")] -> w273
          frame "in range", Default {
            # "right wing"
            n107 = Subtract(x=w294, y=w290) -> (x-y=w289:dbl)
            n108 = Divide(x=w289, y=w293) -> (x/y=w292:dbl)
            n109 = Multiply(x=w292, y=w291) -> (x*y=w288:dbl)
            n110 = Subtract(x=w290, y=w288) -> (x-y=w286:dbl)
            n111 = Add(x=w289, y=w290) -> (x+y=w287:dbl)
          }
          frame "below" {
            # "right wing"
            # "left wing"
            n112 = Subtract(x=w297, y=w296) -> (x-y=w301:dbl)
            n113 = Divide(x=w301, y=w304) -> (x/y=w303:dbl)
            n114 = Multiply(x=w303, y=w302) -> (x*y=w299:dbl)
            n115 = Subtract(x=w297, y=w301) -> (x-y=w300:dbl)
            n116 = Add(x=w299, y=w297) -> (x+y=w298:dbl)
          }
        }
        n117 = Bundle By Name(cluster=w281, "left"=w283, "right"=w284, "window"=w282, "wing order"=w273) -> (w271:T1)
      }
      frame "-set center.Y" {
        # "zero"
        # "calculate center.Y   from"
        # "complementary to calculation of fraction from vert offset"
        n118 = Unbundle By Name(w322) -> ("scale.y.halfwidth"=w319:dbl, "scale.y.center"=w320:dbl, "scale.x.range"=w326:dbl, "scale.y.max"=w325:dbl, "scale.y.min"=w324:dbl)
        n119 = Unbundle By Name(w316) -> ("window"=w327:dbl, "fixed vertical offset"=w328:dbl, "kind"=w306:enum16{"symmetric", "skewed", "fancy"}, "default window frac"=w329:dbl, "skew"=w305:dbl)
        n120 = case shown="\"symmetric\", Default" w306 {
          tunnel: w329 -> [w341 _]
          tunnel: w327 -> [w340 _]
          tunnel: w326 -> [w339 _]
          tunnel: [w330 w342] -> w307
          tunnel: w305 -> [_ w342]
          frame "symmetric", Default {
            # "window fraction"
            # "-1..1"
            n121 = Multiply(x=w339, y=w341) -> (x*y=w335:dbl)
            n122 = Divide(x=w340, y=w335) -> (x/y=w334:dbl)
            n123 = call "Q -- check range -- i -- real.vi"("upper"=0.99 ("y"), "lower"=0.0 ("y"), "number"=w334) -> ("number in range"=w331:dbl)  [unwired: 6 in, 2 out]
            n124 = Multiply(x=2.0, y=w331) -> (x*y=w338:dbl)
            n125 = Subtract(x=w338, y=1.0) -> (x-y=w330:dbl)
          }
          frame "skewed" {
          }
        }
        n126 = Multiply(x=w328, y=1.0) -> (x*y=w310:dbl)
        n127 = Multiply(x=w310, y=w319) -> (x*y=w315:dbl)
        n128 = Add(x=w320, y=w315) -> (x+y=w308:dbl)
        n129 = Subtract(x=w308, y=w324) -> (x-y=w313:dbl)
        n130 = Subtract(x=w325, y=w308) -> (x-y=w314:dbl)
        n131 = Max & Min(x=w314, y=w313) -> (min(x,y)=w312:dbl)  [unwired: 1 out]
        n132 = Multiply(x=w312, y=w307) -> (x*y=w309:dbl)
        n133 = Add(x=w308, y=w309) -> (x+y=w323:dbl)
        n134 = Bundle By Name(cluster=w322, "center.Y"=w323) -> (w321:T3)
      }
      frame "cursor moves" {
        n135 = Unbundle By Name(w355) -> ("cursors"=w354:i32[], "kind"=w345:enum16{"symmetric", "skewed", "fancy"})
        n136 = case shown="\"fancy\"" w345 {
          tunnel: [w357 w361] -> w344
          tunnel: w343 -> [w357 w360]
          frame "symmetric", Default {
          }
          frame "fancy" {
            n137 = call "cursor window action stack.vi"("stack action"=stack_action_--_control."push", "cursor window action"=cursor_window_action."-write plot scale", "command stack"=w360) -> ("command stack out"=w361:T2[])  [unwired: 6 in, 2 out]
          }
        }
        n138 = Array Max & Min(array=w354) -> (max value=w352:i32, min value=w351:i32)  [unwired: 2 out]
        n139 = call "Q -- check range -- i -- integer.vi"("upper"=w352, "lower"=w351, "number"=w346) -> ("in range?"=w350:bool)  [unwired: 6 in, 2 out]
        n140 = Subtract(x=w346, y=w351) -> (x-y=w353:i32)
        n141 = case shown="True" w350 {
          tunnel: w344 -> [w363 w370]
          tunnel: [w363 w369] -> w356
          tunnel: w355 -> [w362 w368]
          tunnel: [w362 w367] -> w347
          tunnel: w354 -> [_ w366]
          tunnel: w353 -> [_ w365]
          frame False {
          }
          frame True {
            n142 = Index Array(array=w366, index=w365) -> (element=w364:i32)
            n143 = Bundle By Name(cluster=w368, "absolute"=w364, "relative"=w365) -> (w367:T1)
            n144 = case shown="0, 2, Default" w365 {
              selector: w365 -> [_ w380]
              tunnel: w370 -> [w374 w382]
              tunnel: [w373 w381] -> w369
              frame 1 {
                w371 = T2[] [enum."-read cursor 1", enum."-read plot scale", enum."-parse center.Y", enum."-copy cursor 1", enum."-change center", enum."-write right.X", enum."-write left.X"] items=["balance", "h. offset change", "cursor moves", "change center", "change window", "init", "check", "reset", "set y to middle", "idle", "-write all Y", "-write left.X", "-write center.X", "-write right.X", "-write all X", "-change center", "-change window", "-change skew", "-read cursor 2", "-read cursor 1", "-read cursor 0", "-read all cursors", "-reset", "-read plot scale", "-set y to middle", "-Q: center.Y is visible", "-Q: window is visible", "-parse center.Y", "-right left from center", "-left move", "-right move", "-set center.Y", "-empty", "-set cursors to default", "-check", "-write center.Y", "-copy cursor 1", "-copy cursor 0", "-copy cursor 2", "move right", "move left", "shrink", "broaden", "skew up", "skew down", "-write plot scale", "zoom X", "change cen&win", "zoom to all data", "color--red", "color--green", "color--yellow", "read", "zoom out", "zoom in", "slide right", "slide left", "set range aspect ratio to 1"]
                n145 = call "cursor window action stack.vi"("stack action"=stack_action_--_control."push", "action list"=w371, "command stack"=w374) -> ("command stack out"=w373:T2[])  [unwired: 6 in, 2 out]
              }
              frame 0, 2, Default {
                w379 = T2[] [enum."-set center.Y", enum."-write center.Y"] items=["balance", "h. offset change", "cursor moves", "change center", "change window", "init", "check", "reset", "set y to middle", "idle", "-write all Y", "-write left.X", "-write center.X", "-write right.X", "-write all X", "-change center", "-change window", "-change skew", "-read cursor 2", "-read cursor 1", "-read cursor 0", "-read all cursors", "-reset", "-read plot scale", "-set y to middle", "-Q: center.Y is visible", "-Q: window is visible", "-parse center.Y", "-right left from center", "-left move", "-right move", "-set center.Y", "-empty", "-set cursors to default", "-check", "-write center.Y", "-copy cursor 1", "-copy cursor 0", "-copy cursor 2", "move right", "move left", "shrink", "broaden", "skew up", "skew down", "-write plot scale", "zoom X", "change cen&win", "zoom to all data", "color--red", "color--green", "color--yellow", "read", "zoom out", "zoom in", "slide right", "slide left", "set range aspect ratio to 1"]
                w377 = T2[] [enum."-read plot scale"] items=["balance", "h. offset change", "cursor moves", "change center", "change window", "init", "check", "reset", "set y to middle", "idle", "-write all Y", "-write left.X", "-write center.X", "-write right.X", "-write all X", "-change center", "-change window", "-change skew", "-read cursor 2", "-read cursor 1", "-read cursor 0", "-read all cursors", "-reset", "-read plot scale", "-set y to middle", "-Q: center.Y is visible", "-Q: window is visible", "-parse center.Y", "-right left from center", "-left move", "-right move", "-set center.Y", "-empty", "-set cursors to default", "-check", "-write center.Y", "-copy cursor 1", "-copy cursor 0", "-copy cursor 2", "move right", "move left", "shrink", "broaden", "skew up", "skew down", "-write plot scale", "zoom X", "change cen&win", "zoom to all data", "color--red", "color--green", "color--yellow", "read", "zoom out", "zoom in", "slide right", "slide left", "set range aspect ratio to 1"]
                n146 = case shown="0, Default" w380 {
                  tunnel: [w383 w384] -> w378
                  frame 0, Default {
                    w383 = T2[] [enum."-read cursor 0", enum."-left move", enum."-write right.X"] items=["balance", "h. offset change", "cursor moves", "change center", "change window", "init", "check", "reset", "set y to middle", "idle", "-write all Y", "-write left.X", "-write center.X", "-write right.X", "-write all X", "-change center", "-change window", "-change skew", "-read cursor 2", "-read cursor 1", "-read cursor 0", "-read all cursors", "-reset", "-read plot scale", "-set y to middle", "-Q: center.Y is visible", "-Q: window is visible", "-parse center.Y", "-right left from center", "-left move", "-right move", "-set center.Y", "-empty", "-set cursors to default", "-check", "-write center.Y", "-copy cursor 1", "-copy cursor 0", "-copy cursor 2", "move right", "move left", "shrink", "broaden", "skew up", "skew down", "-write plot scale", "zoom X", "change cen&win", "zoom to all data", "color--red", "color--green", "color--yellow", "read", "zoom out", "zoom in", "slide right", "slide left", "set range aspect ratio to 1"]
                  }
                  frame 2 {
                    w384 = T2[] [enum."-read cursor 2", enum."-right move", enum."-write left.X"] items=["balance", "h. offset change", "cursor moves", "change center", "change window", "init", "check", "reset", "set y to middle", "idle", "-write all Y", "-write left.X", "-write center.X", "-write right.X", "-write all X", "-change center", "-change window", "-change skew", "-read cursor 2", "-read cursor 1", "-read cursor 0", "-read all cursors", "-reset", "-read plot scale", "-set y to middle", "-Q: center.Y is visible", "-Q: window is visible", "-parse center.Y", "-right left from center", "-left move", "-right move", "-set center.Y", "-empty", "-set cursors to default", "-check", "-write center.Y", "-copy cursor 1", "-copy cursor 0", "-copy cursor 2", "move right", "move left", "shrink", "broaden", "skew up", "skew down", "-write plot scale", "zoom X", "change cen&win", "zoom to all data", "color--red", "color--green", "color--yellow", "read", "zoom out", "zoom in", "slide right", "slide left", "set range aspect ratio to 1"]
                  }
                }
                n147 = Build Array (concatenate)(w377, w378, w379) -> (w375:T2[])
                n148 = call "cursor window action stack.vi"("stack action"=stack_action_--_control."push", "action list"=w375, "command stack"=w382) -> ("command stack out"=w381:T2[])  [unwired: 6 in, 2 out]
              }
            }
          }
        }
      }
      frame "idle" {
        n149 = disable-structure shown="Disabled" {
          frame Disabled {
            w389 = "win:left"  # Name
            w395 = u32 0  # Cursor Mode
            w394 = TRUE  # Allow Drag
            w393 = FALSE  # Name Visible
            w392 = u8 0  # Point Style
            w391 = u8 2  # Style
            n150 = Bundle By Name("Name"=w389, "Color"=u32 16768256, "Style"=w391, "Point Style"=w392, "Name Visible"=w393, "Allow Drag"=w394, "Cursor Mode"=w395) -> ()  [unwired: 1 in, 1 out]
            n151 = call "Q -- check range -- i -- real.vi"() -> ()  [unwired: 9 in, 3 out]
          }
          frame Enabled {
          }
        }
      }
      frame "-copy cursor 1" {
        n152 = Unbundle By Name(w401) -> ("center.X"=w400:dbl)
        n153 = Bundle By Name(cluster=w398, "center"=w400) -> (w397:T1)
      }
      frame "-set y to middle" {
        w402 = 0.5
        n154 = Unbundle By Name(w405) -> ("fixed vertical offset"=w411:dbl)
        n155 = Unbundle By Name(w410) -> ("scale.y.center"=w406:dbl, "scale.y.halfwidth"=w407:dbl)
        n156 = Multiply(x=w407, y=w411) -> (x*y=w412:dbl)
        n157 = Bundle By Name(cluster=w405, "skew"=0.0, "skew.left"=w402, "skew.right"=w402) -> (w404:T1)
        n158 = Add(x=w406, y=w412) -> (x+y=w408:dbl)
        n159 = Bundle By Name(cluster=w410, "right.Y"=w408, "center.Y"=w408, "left.Y"=w408) -> (w409:T3)
      }
      frame "-set cursors to default" {
        w418 = 0.5
        w417 = 0.1
        (unwired) 3
        n160 = Unbundle By Name(w428) -> ("scale.x.halfwidth"=w416:dbl, "scale.x.center"=w422:dbl)
        n161 = Multiply(x=w416, y=w417) -> (x*y=w415:dbl)
        n162 = Multiply(x=w415, y=2) -> (x*y=w421:dbl)
        n163 = Add(x=w422, y=w415) -> (x+y=w426:dbl)
        n164 = Subtract(x=w422, y=w415) -> (x-y=w427:dbl)
        n165 = Bundle By Name(cluster=w424, "vertical offset"=0.0, "default window frac"=w417, "left"=w427, "right"=w426, "center"=w422, "window"=w421, "skew"=0.0, "skew.left"=w418, "skew.right"=w418) -> (w420:T1)
      }
      frame "-read plot scale" {
        w441 = 2.0 ("y")
        w446 = 2.0 ("y")
        n166 = Unbundle By Name(w437) -> ("Plot ref"=w436:refnum<vi>)
        n167 = call "replace cursor - plot ref - V2.vi"("Plot ref in"=w436) -> ("2Dwindow bounds out"=w435:T12)  [unwired: 15 in, 3 out]
        n168 = Unbundle By Name(w435) -> ("max y"=w434:dbl, "min y"=w433:dbl, "max x"=w432:dbl, "min x"=w431:dbl)
        n169 = Add(x=w432, y=w431) -> (x+y=w447:dbl)
        n170 = Subtract(x=w432, y=w431) -> (x-y=w445:dbl)
        n171 = Divide(x=w447, y=w446) -> (x/y=w444:dbl)
        n172 = Divide(x=w445, y=w446) -> (x/y=w443:dbl)
        n173 = Subtract(x=w434, y=w433) -> (x-y=w438:dbl)
        n174 = Add(x=w434, y=w433) -> (x+y=w442:dbl)
        n175 = Divide(x=w442, y=w441) -> (x/y=w440:dbl)
        n176 = Divide(x=w438, y=w441) -> (x/y=w439:dbl)
        n177 = Bundle By Name(cluster=w450, "scale.y.max"=w434, "scale.y.min"=w433, "scale.x.max"=w432, "scale.x.min"=w431, "scale.x.range"=w445, "scale.x.halfwidth"=w443, "scale.x.center"=w444, "scale.y.range"=w438, "scale.y.halfwidth"=w439, "scale.y.center"=w440) -> (w449:T3)
      }
      frame "-write plot scale" {
        n178 = Unbundle By Name(w463) -> ("Plot ref"=w456:refnum<vi>, "window"=w460:dbl, "center"=w459:dbl, "default window frac"=w458:dbl)
        n179 = call "Q -- range multiplier -- real -- V2.vi"("factor"=w458, "rage multiplier action"=range_multiplier_action."zoom", "center"=w459, "window"=w460) -> ("center OUT"=w454:dbl, "window OUT"=w453:dbl)  [unwired: 4 in, 2 out]
        n180 = Bundle By Name(cluster=T9 {"window y"=0.0021014740628288917, "center x"=44850.89441339177, "center y"=2.5658109925320947, "window x"=17480.201988350764} ("window IN"), "window x"=w453, "center x"=w454) -> (w452:T9)
        n181 = call "replace cursor - plot ref - V2.vi"("Plot ref in"=w456, "window IN"=w452, "cursor action"=cursor_action."zoom to X win") -> ()  [unwired: 13 in, 4 out]
      }
      frame "zoom X" {
        n182 = Unbundle By Name(w478) -> ("Plot ref"=w470:refnum<vi>, "window"=w469:dbl, "center"=w468:dbl, "default window frac"=w467:dbl)
        n183 = Reciprocal(x=w467) -> (1/x=w466:dbl)
        n184 = call "Q -- range multiplier -- real -- V2.vi"("factor"=w466, "rage multiplier action"=range_multiplier_action."zoom", "center"=w468, "window"=w469) -> ("center OUT"=w473:dbl, "window OUT"=w472:dbl)  [unwired: 4 in, 2 out]
        n185 = Bundle By Name(cluster=T9 {"window y"=0.0021014740628288917, "center x"=44850.89441339177, "center y"=2.5658109925320947, "window x"=17480.201988350764} ("window IN"), "window x"=w472, "center x"=w473) -> (w471:T9)
        n186 = call "replace cursor - plot ref - V2.vi"("Plot ref in"=w470, "window IN"=w471, "cursor action"=cursor_action."zoom to X win") -> ()  [unwired: 13 in, 4 out]
      }
      frame "zoom out" {
        (unwired) range_multiplier_action."zoom" ("rage multiplier action")
        n187 = Unbundle By Name(w484) -> ("Plot ref"=w481:refnum<vi>)
        n188 = call "replace cursor - plot ref - V2.vi"("Plot ref in"=w481, "cursor action"=cursor_action."zoom out X") -> ()  [unwired: 14 in, 4 out]
      }
      frame "set range aspect ratio to 1" {
        n189 = Unbundle By Name(w490) -> ("Plot ref"=w488:refnum<vi>)
        n190 = call "replace cursor - plot ref - V2.vi"("Plot ref in"=w488, "cursor action"=cursor_action."zoom to aspect ratio 1") -> ()  [unwired: 14 in, 4 out]
      }
      frame "zoom in" {
        n191 = Unbundle By Name(w496) -> ("Plot ref"=w494:refnum<vi>)
        n192 = call "replace cursor - plot ref - V2.vi"("Plot ref in"=w494, "cursor action"=cursor_action."zoom in X") -> ()  [unwired: 14 in, 4 out]
      }
      frame "slide right" {
        n193 = Unbundle By Name(w502) -> ("Plot ref"=w500:refnum<vi>)
        n194 = call "replace cursor - plot ref - V2.vi"("Plot ref in"=w500, "cursor action"=cursor_action."move range right 20%") -> ()  [unwired: 14 in, 4 out]
      }
      frame "slide left" {
        n195 = Unbundle By Name(w508) -> ("Plot ref"=w506:refnum<vi>)
        n196 = call "replace cursor - plot ref - V2.vi"("Plot ref in"=w506, "cursor action"=cursor_action."move range left 20%") -> ()  [unwired: 14 in, 4 out]
      }
      frame "-Q: center.Y is visible" {
        # "check if y is within y-scale bounds"
        n197 = Unbundle By Name(w517) -> ("center.Y"=w520:dbl, "scale.y.max"=w519:dbl, "scale.y.min"=w518:dbl, "scale.y.center"=w511:dbl)
        n198 = call "Q -- check range -- i -- real.vi"("upper"=w519, "lower"=w518, "number"=w520) -> ("in range?"=w512:bool)  [unwired: 6 in, 2 out]
        n199 = case shown="False" w512 {
          tunnel: w517 -> [w528 w530]
          tunnel: [w527 w530] -> w516
          tunnel: w514 -> [w525 w529]
          tunnel: [w523 w529] -> w513
          tunnel: w511 -> [w522 _]
          frame False {
            w526 = T2[] [enum."-parse center.Y", enum."-write center.Y"] items=["balance", "h. offset change", "cursor moves", "change center", "change window", "init", "check", "reset", "set y to middle", "idle", "-write all Y", "-write left.X", "-write center.X", "-write right.X", "-write all X", "-change center", "-change window", "-change skew", "-read cursor 2", "-read cursor 1", "-read cursor 0", "-read all cursors", "-reset", "-read plot scale", "-set y to middle", "-Q: center.Y is visible", "-Q: window is visible", "-parse center.Y", "-right left from center", "-left move", "-right move", "-set center.Y", "-empty", "-set cursors to default", "-check", "-write center.Y", "-copy cursor 1", "-copy cursor 0", "-copy cursor 2", "move right", "move left", "shrink", "broaden", "skew up", "skew down", "-write plot scale", "zoom X", "change cen&win", "zoom to all data", "color--red", "color--green", "color--yellow", "read", "zoom out", "zoom in", "slide right", "slide left", "set range aspect ratio to 1"]
            n200 = Bundle By Name(cluster=w528, "center.Y"=w522) -> (w527:T3)
            n201 = call "cursor window action stack.vi"("stack action"=stack_action_--_control."push", "action list"=w526, "command stack"=w525) -> ("command stack out"=w523:T2[])  [unwired: 6 in, 2 out]
          }
          frame True {
          }
        }
      }
      frame "move left" {
        (unwired) 0.2
        w543 = T2[] [enum."-change center", enum."-write all X"] items=["balance", "h. offset change", "cursor moves", "change center", "change window", "init", "check", "reset", "set y to middle", "idle", "-write all Y", "-write left.X", "-write center.X", "-write right.X", "-write all X", "-change center", "-change window", "-change skew", "-read cursor 2", "-read cursor 1", "-read cursor 0", "-read all cursors", "-reset", "-read plot scale", "-set y to middle", "-Q: center.Y is visible", "-Q: window is visible", "-parse center.Y", "-right left from center", "-left move", "-right move", "-set center.Y", "-empty", "-set cursors to default", "-check", "-write center.Y", "-copy cursor 1", "-copy cursor 0", "-copy cursor 2", "move right", "move left", "shrink", "broaden", "skew up", "skew down", "-write plot scale", "zoom X", "change cen&win", "zoom to all data", "color--red", "color--green", "color--yellow", "read", "zoom out", "zoom in", "slide right", "slide left", "set range aspect ratio to 1"]
        n202 = Unbundle By Name(w539) -> ("center"=w533:dbl, "window"=w532:dbl, "default window frac"=w531:dbl)  [unwired: 1 out]
        n203 = Multiply(x=w532, y=w531) -> (x*y=w534:dbl)
        n204 = Subtract(x=w533, y=w534) -> (x-y=w537:dbl)
        n205 = Bundle By Name(cluster=w539, "center"=w537) -> (w538:T1)
        n206 = call "cursor window action stack.vi"("stack action"=stack_action_--_control."push", "action list"=w543, "command stack"=w541) -> ("command stack out"=w540:T2[])  [unwired: 6 in, 2 out]
      }
      frame "move right" {
        (unwired) 0.2
        w556 = T2[] [enum."-change center", enum."-write all X"] items=["balance", "h. offset change", "cursor moves", "change center", "change window", "init", "check", "reset", "set y to middle", "idle", "-write all Y", "-write left.X", "-write center.X", "-write right.X", "-write all X", "-change center", "-change window", "-change skew", "-read cursor 2", "-read cursor 1", "-read cursor 0", "-read all cursors", "-reset", "-read plot scale", "-set y to middle", "-Q: center.Y is visible", "-Q: window is visible", "-parse center.Y", "-right left from center", "-left move", "-right move", "-set center.Y", "-empty", "-set cursors to default", "-check", "-write center.Y", "-copy cursor 1", "-copy cursor 0", "-copy cursor 2", "move right", "move left", "shrink", "broaden", "skew up", "skew down", "-write plot scale", "zoom X", "change cen&win", "zoom to all data", "color--red", "color--green", "color--yellow", "read", "zoom out", "zoom in", "slide right", "slide left", "set range aspect ratio to 1"]
        n207 = Unbundle By Name(w545) -> ("center"=w548:dbl, "window"=w547:dbl, "default window frac"=w546:dbl)  [unwired: 1 out]
        n208 = Multiply(x=w547, y=w546) -> (x*y=w549:dbl)
        n209 = Add(x=w548, y=w549) -> (x+y=w550:dbl)
        n210 = Bundle By Name(cluster=w545, "center"=w550) -> (w544:T1)
        n211 = call "cursor window action stack.vi"("stack action"=stack_action_--_control."push", "action list"=w556, "command stack"=w554) -> ("command stack out"=w553:T2[])  [unwired: 6 in, 2 out]
      }
      frame "shrink" {
        (unwired) 0.3
        w569 = T2[] [enum."-change window", enum."-write all X", enum."-read plot scale", enum."-set center.Y", enum."-write center.Y"] items=["balance", "h. offset change", "cursor moves", "change center", "change window", "init", "check", "reset", "set y to middle", "idle", "-write all Y", "-write left.X", "-write center.X", "-write right.X", "-write all X", "-change center", "-change window", "-change skew", "-read cursor 2", "-read cursor 1", "-read cursor 0", "-read all cursors", "-reset", "-read plot scale", "-set y to middle", "-Q: center.Y is visible", "-Q: window is visible", "-parse center.Y", "-right left from center", "-left move", "-right move", "-set center.Y", "-empty", "-set cursors to default", "-check", "-write center.Y", "-copy cursor 1", "-copy cursor 0", "-copy cursor 2", "move right", "move left", "shrink", "broaden", "skew up", "skew down", "-write plot scale", "zoom X", "change cen&win", "zoom to all data", "color--red", "color--green", "color--yellow", "read", "zoom out", "zoom in", "slide right", "slide left", "set range aspect ratio to 1"]
        n212 = Unbundle By Name(w565) -> ("window"=w560:dbl, "window"=w559:dbl, "default window frac"=w557:dbl)
        n213 = Multiply(x=w559, y=w557) -> (x*y=w558:dbl)
        n214 = Subtract(x=w560, y=w558) -> (x-y=w563:dbl)
        n215 = Bundle By Name(cluster=w565, "window"=w563) -> (w564:T1)
        n216 = call "cursor window action stack.vi"("stack action"=stack_action_--_control."push", "action list"=w569, "command stack"=w567) -> ("command stack out"=w566:T2[])  [unwired: 6 in, 2 out]
      }
      frame "broaden" {
        (unwired) 0.3
        w577 = T2[] [enum."-change window", enum."-write all X", enum."-read plot scale", enum."-set center.Y", enum."-write center.Y"] items=["balance", "h. offset change", "cursor moves", "change center", "change window", "init", "check", "reset", "set y to middle", "idle", "-write all Y", "-write left.X", "-write center.X", "-write right.X", "-write all X", "-change center", "-change window", "-change skew", "-read cursor 2", "-read cursor 1", "-read cursor 0", "-read all cursors", "-reset", "-read plot scale", "-set y to middle", "-Q: center.Y is visible", "-Q: window is visible", "-parse center.Y", "-right left from center", "-left move", "-right move", "-set center.Y", "-empty", "-set cursors to default", "-check", "-write center.Y", "-copy cursor 1", "-copy cursor 0", "-copy cursor 2", "move right", "move left", "shrink", "broaden", "skew up", "skew down", "-write plot scale", "zoom X", "change cen&win", "zoom to all data", "color--red", "color--green", "color--yellow", "read", "zoom out", "zoom in", "slide right", "slide left", "set range aspect ratio to 1"]
        n217 = Unbundle By Name(w571) -> ("window"=w575:dbl, "window"=w574:dbl, "default window frac"=w572:dbl)
        n218 = Multiply(x=w574, y=w572) -> (x*y=w573:dbl)
        n219 = Add(x=w575, y=w573) -> (x+y=w576:dbl)
        n220 = Bundle By Name(cluster=w571, "window"=w576) -> (w570:T1)
        n221 = call "cursor window action stack.vi"("stack action"=stack_action_--_control."push", "action list"=w577, "command stack"=w581) -> ("command stack out"=w580:T2[])  [unwired: 6 in, 2 out]
      }
      frame "skew up" {
        n222 = Unbundle By Name(w584) -> ("kind"=w583:enum16{"symmetric", "skewed", "fancy"})
        n223 = case shown="\"skewed\"" w583 {
          tunnel: w589 -> [w591 w601]
          tunnel: [w591 w600] -> w588
          tunnel: [w590 w599] -> w587
          tunnel: w584 -> [w590 w597]
          frame "symmetric", Default {
          }
          frame "skewed" {
            w603 = T2[] [enum."-change skew", enum."-read plot scale", enum."-set center.Y", enum."-write right.X", enum."-write left.X", enum."-write center.Y"] items=["balance", "h. offset change", "cursor moves", "change center", "change window", "init", "check", "reset", "set y to middle", "idle", "-write all Y", "-write left.X", "-write center.X", "-write right.X", "-write all X", "-change center", "-change window", "-change skew", "-read cursor 2", "-read cursor 1", "-read cursor 0", "-read all cursors", "-reset", "-read plot scale", "-set y to middle", "-Q: center.Y is visible", "-Q: window is visible", "-parse center.Y", "-right left from center", "-left move", "-right move", "-set center.Y", "-empty", "-set cursors to default", "-check", "-write center.Y", "-copy cursor 1", "-copy cursor 0", "-copy cursor 2", "move right", "move left", "shrink", "broaden", "skew up", "skew down", "-write plot scale", "zoom X", "change cen&win", "zoom to all data", "color--red", "color--green", "color--yellow", "read", "zoom out", "zoom in", "slide right", "slide left", "set range aspect ratio to 1"]
            n224 = Unbundle By Name(w597) -> ("skew"=w598:dbl)
            n225 = Add(x=0.1, y=w598) -> (x+y=w595:dbl)
            n226 = call "Q -- check range -- i -- real.vi"("upper"=1, "lower"=-1, "number"=w595) -> ("number in range"=w592:dbl)  [unwired: 6 in, 2 out]
            n227 = Bundle By Name(cluster=w597, "skew"=w592) -> (w599:T1)
            n228 = call "cursor window action stack.vi"("stack action"=stack_action_--_control."push", "action list"=w603, "command stack"=w601) -> ("command stack out"=w600:T2[])  [unwired: 6 in, 2 out]
          }
        }
      }
      frame "skew down" {
        n229 = Unbundle By Name(w605) -> ("kind"=w604:enum16{"symmetric", "skewed", "fancy"})
        n230 = case shown="\"skewed\"" w604 {
          tunnel: w610 -> [w612 w623]
          tunnel: [w612 w622] -> w609
          tunnel: [w611 w621] -> w608
          tunnel: w605 -> [w611 w620]
          frame "symmetric", Default {
          }
          frame "skewed" {
            w615 = T2[] [enum."-change skew", enum."-read plot scale", enum."-set center.Y", enum."-write right.X", enum."-write left.X", enum."-write center.Y"] items=["balance", "h. offset change", "cursor moves", "change center", "change window", "init", "check", "reset", "set y to middle", "idle", "-write all Y", "-write left.X", "-write center.X", "-write right.X", "-write all X", "-change center", "-change window", "-change skew", "-read cursor 2", "-read cursor 1", "-read cursor 0", "-read all cursors", "-reset", "-read plot scale", "-set y to middle", "-Q: center.Y is visible", "-Q: window is visible", "-parse center.Y", "-right left from center", "-left move", "-right move", "-set center.Y", "-empty", "-set cursors to default", "-check", "-write center.Y", "-copy cursor 1", "-copy cursor 0", "-copy cursor 2", "move right", "move left", "shrink", "broaden", "skew up", "skew down", "-write plot scale", "zoom X", "change cen&win", "zoom to all data", "color--red", "color--green", "color--yellow", "read", "zoom out", "zoom in", "slide right", "slide left", "set range aspect ratio to 1"]
            n231 = Unbundle By Name(w620) -> ("skew"=w614:dbl)
            n232 = Subtract(x=w614, y=0.1) -> (x-y=w619:dbl)
            n233 = call "Q -- check range -- i -- real.vi"("upper"=1, "lower"=-1, "number"=w619) -> ("number in range"=w616:dbl)  [unwired: 6 in, 2 out]
            n234 = Bundle By Name(cluster=w620, "skew"=w616) -> (w621:T1)
            n235 = call "cursor window action stack.vi"("stack action"=stack_action_--_control."push", "action list"=w615, "command stack"=w623) -> ("command stack out"=w622:T2[])  [unwired: 6 in, 2 out]
          }
        }
      }
      frame "-parse center.Y" {
        w637 = 1.0  # y
        w639 = 2.0  # y
        # "left factor"
        # "right factor"
        # "0 .. 1"
        # "-1 .. 1"
        # "-1..1"
        # "\"zero\""
        # "calculate horizontal offset and/or window \nfrom vertical position of center cursor"
        n236 = Unbundle By Name(w648) -> ("center.Y"=w633:dbl, "scale.y.max"=w631:dbl, "scale.y.min"=w632:dbl, "scale.y.center"=w629:dbl, "scale.y.halfwidth"=w641:dbl)
        n237 = Unbundle By Name(w644) -> ("fixed vertical offset"=w661:dbl)
        n238 = Multiply(x=w641, y=w661) -> (x*y=w659:dbl)
        n239 = call "Q -- check range -- i -- real.vi"("upper"=w631, "lower"=w632, "default"=w629, "number"=w633) -> ("number in range"=w630:dbl)  [unwired: 5 in, 2 out]
        n240 = Add(x=w659, y=w629) -> (x+y=w656:dbl)
        n241 = Unbundle By Name(w644) -> ("default window frac"=w649:dbl, "kind"=w650:enum16{"symmetric", "skewed", "fancy"}, "skew"=w646:dbl, "window"=w645:dbl)
        n242 = Unbundle By Name(w648) -> ("scale.x.range"=w647:dbl)
        n243 = Subtract(x=w656, y=w632) -> (x-y=w657:dbl)
        n244 = Subtract(x=w631, y=w656) -> (x-y=w658:dbl)
        n245 = Max & Min(x=w658, y=w657) -> (min(x,y)=w654:dbl)  [unwired: 1 out]
        n246 = Subtract(x=w630, y=w656) -> (x-y=w655:dbl)
        n247 = Divide(x=w655, y=w654) -> (x/y=w653:dbl)
        n248 = Multiply(x=w653, y=0.99) -> (x*y=w628:dbl)
        n249 = call "Q -- check range -- i -- real.vi"("upper"=1, "lower"=-1, "number"=w628) -> ("number in range"=w625:dbl)  [unwired: 6 in, 2 out]
        n250 = Bundle By Name(cluster=w648, "center.Y"=w630) -> (w651:T3)
        n251 = case shown="\"symmetric\", Default" w650 {
          tunnel: [w662 w673] -> w636
          tunnel: w625 -> [w671 w673]
          tunnel: w649 -> [w670 _]
          tunnel: w647 -> [w669 _]
          tunnel: [w663 w672] -> w643
          tunnel: w646 -> [w662 _]
          tunnel: w645 -> [_ w672]
          frame "symmetric", Default {
            # "0 .. 1"
            # "-1 .. 1"
            n252 = Add(x=w671, y=1.0) -> (x+y=w667:dbl)
            n253 = Divide(x=w667, y=2.0) -> (x/y=w665:dbl)
            n254 = Multiply(x=w670, y=w665) -> (x*y=w664:dbl)
            n255 = Multiply(x=w664, y=w669) -> (x*y=w663:dbl)
          }
          frame "skewed" {
          }
        }
        n256 = Add(x=w636, y=w637) -> (x+y=w638:dbl)
        n257 = Divide(x=w638, y=w639) -> (x/y=w634:dbl)
        n258 = Subtract(x=w637, y=w634) -> (x-y=w635:dbl)
        n259 = Bundle By Name(cluster=w644, "skew"=w636, "window"=w643, "skew.left"=w635, "skew.right"=w634) -> (w640:T1)
      }
      frame "-Q: window is visible" {
        n260 = Unbundle By Name(w684) -> ("scale.x.min"=w676:dbl, "scale.x.max"=w675:dbl, "scale.x.center"=w679:dbl, "scale.x.range"=w674:dbl)  [unwired: 1 out]
        n261 = Unbundle By Name(w678) -> ("center"=w683:dbl)
        n262 = call "Q -- check range -- i -- real.vi"("upper"=w675, "lower"=w676, "number"=w683) -> ("selector"=w682:T11)  [unwired: 6 in, 2 out]
        n263 = case shown="\"in range\"" w682 {
          tunnel: w681 -> [w691 w716]
          tunnel: [w690 w714] -> w680
          tunnel: w678 -> [w689 w713]
          tunnel: w679 -> [_ w712]
          tunnel: [w687 w711] -> w677
          tunnel: w676 -> [w697 _]
          tunnel: w675 -> [w696 _]
          tunnel: w674 -> [w688 _]
          frame "in range" {
            n264 = Unbundle By Name(w689) -> ("left"=w699:dbl, "right"=w698:dbl)
            n265 = call "Q -- check range -- i -- real.vi"("upper"=w696, "lower"=w697, "number"=w699) -> ("in range?"=w695:bool)  [unwired: 6 in, 2 out]
            n266 = call "Q -- check range -- i -- real.vi"("upper"=w696, "lower"=w697, "number"=w698) -> ("in range?"=w694:bool)  [unwired: 6 in, 2 out]
            n267 = Not(x=w695) -> (.not. x?=w693:bool)
            n268 = Not(x=w694) -> (.not. x?=w692:bool)
            n269 = And(x=w693, y=w692) -> (x .and. y?=w686:bool)
            n270 = case shown="True" w686 {
              tunnel: w691 -> [w701 w708]
              tunnel: [w701 w707] -> w690
              tunnel: w689 -> [w700 w706]
              tunnel: w688 -> [_ w704]
              tunnel: [w700 w702] -> w687
              frame False {
              }
              frame True {
                w710 = T2[] [enum."-change window", enum."-write left.X", enum."-write right.X"] items=["balance", "h. offset change", "cursor moves", "change center", "change window", "init", "check", "reset", "set y to middle", "idle", "-write all Y", "-write left.X", "-write center.X", "-write right.X", "-write all X", "-change center", "-change window", "-change skew", "-read cursor 2", "-read cursor 1", "-read cursor 0", "-read all cursors", "-reset", "-read plot scale", "-set y to middle", "-Q: center.Y is visible", "-Q: window is visible", "-parse center.Y", "-right left from center", "-left move", "-right move", "-set center.Y", "-empty", "-set cursors to default", "-check", "-write center.Y", "-copy cursor 1", "-copy cursor 0", "-copy cursor 2", "move right", "move left", "shrink", "broaden", "skew up", "skew down", "-write plot scale", "zoom X", "change cen&win", "zoom to all data", "color--red", "color--green", "color--yellow", "read", "zoom out", "zoom in", "slide right", "slide left", "set range aspect ratio to 1"]
                n271 = Unbundle By Name(w706) -> ("default window frac"=w705:dbl)
                n272 = Multiply(x=w705, y=w704) -> (x*y=w703:dbl)
                n273 = Bundle By Name(cluster=w706, "window"=w703) -> (w702:T1)
                n274 = call "cursor window action stack.vi"("stack action"=stack_action_--_control."push", "action list"=w710, "command stack"=w708) -> ("command stack out"=w707:T2[])  [unwired: 6 in, 2 out]
              }
            }
          }
          frame "not a number", "above", "below", Default {
            w717 = T2[] [enum."-change center", enum."-write all X", enum."-Q: window is visible"] items=["balance", "h. offset change", "cursor moves", "change center", "change window", "init", "check", "reset", "set y to middle", "idle", "-write all Y", "-write left.X", "-write center.X", "-write right.X", "-write all X", "-change center", "-change window", "-change skew", "-read cursor 2", "-read cursor 1", "-read cursor 0", "-read all cursors", "-reset", "-read plot scale", "-set y to middle", "-Q: center.Y is visible", "-Q: window is visible", "-parse center.Y", "-right left from center", "-left move", "-right move", "-set center.Y", "-empty", "-set cursors to default", "-check", "-write center.Y", "-copy cursor 1", "-copy cursor 0", "-copy cursor 2", "move right", "move left", "shrink", "broaden", "skew up", "skew down", "-write plot scale", "zoom X", "change cen&win", "zoom to all data", "color--red", "color--green", "color--yellow", "read", "zoom out", "zoom in", "slide right", "slide left", "set range aspect ratio to 1"]
            n275 = Bundle By Name(cluster=w713, "center"=w712) -> (w711:T1)
            n276 = call "cursor window action stack.vi"("stack action"=stack_action_--_control."push", "action list"=w717, "command stack"=w716) -> ("command stack out"=w714:T2[])  [unwired: 6 in, 2 out]
          }
        }
      }
      frame "-write all X" {
        w734 = cursor_action."write"  # action
        n277 = Unbundle By Name(w718) -> ("Plot ref"=w719:refnum<vi>, "cursors"=w732:i32[], "left"=w726:dbl, "center"=w725:dbl, "right"=w724:dbl)
        n278 = Index Array(array=w732, index #1=0 ("cursor index"), index #2=1 ("cursor index"), index #3=2 ("cursor index")) -> (element #1=w733:i32, element #2=w729:i32, element #3=w727:i32)
        n279 = call "replace cursor - plot ref - V2.vi"("Plot ref in"=w719, "new X"=w726, "cursor index"=w733, "cursor action"=w734) -> ("Plot ref out"=w723:refnum<vi>)  [unwired: 12 in, 3 out]
        n280 = call "replace cursor - plot ref - V2.vi"("Plot ref in"=w723, "new X"=w725, "cursor index"=w729, "cursor action"=w734) -> ("Plot ref out"=w722:refnum<vi>)  [unwired: 12 in, 3 out]
        n281 = call "replace cursor - plot ref - V2.vi"("Plot ref in"=w722, "new X"=w724, "cursor index"=w727, "cursor action"=w734) -> ()  [unwired: 12 in, 4 out]
      }
      frame "color--red" {
        w736 = cursor_sate."colored" ("cursor state")
        w737 = u32 16728794 ("Color Box")
        w738 = cursor_action."write"  # action
        n282 = Unbundle By Name(w739) -> ("Plot ref"=w740:refnum<vi>, "cursors"=w753:i32[], "left"=w747:dbl, "center"=w746:dbl, "right"=w745:dbl)
        n283 = Index Array(array=w753, index #1=0 ("cursor index"), index #2=1 ("cursor index"), index #3=2 ("cursor index")) -> (element #1=w754:i32, element #2=w750:i32, element #3=w748:i32)
        n284 = call "replace cursor - plot ref - V2.vi"("Plot ref in"=w740, "new X"=w747, "cursor index"=w754, "cursor action"=w738, "Color Box"=w737, "cursor state"=w736) -> ("Plot ref out"=w744:refnum<vi>)  [unwired: 10 in, 3 out]
        n285 = call "replace cursor - plot ref - V2.vi"("Plot ref in"=w744, "new X"=w746, "cursor index"=w750, "cursor action"=w738, "Color Box"=w737, "cursor state"=w736) -> ("Plot ref out"=w743:refnum<vi>)  [unwired: 10 in, 3 out]
        n286 = call "replace cursor - plot ref - V2.vi"("Plot ref in"=w743, "new X"=w745, "cursor index"=w748, "cursor action"=w738, "Color Box"=w737, "cursor state"=w736) -> ()  [unwired: 10 in, 4 out]
      }
      frame "color--green" {
        w756 = cursor_sate."colored" ("cursor state")
        w757 = u32 4250624 ("Color Box")
        w758 = cursor_action."write"  # action
        n287 = Unbundle By Name(w759) -> ("Plot ref"=w760:refnum<vi>, "cursors"=w773:i32[], "left"=w767:dbl, "center"=w766:dbl, "right"=w765:dbl)
        n288 = Index Array(array=w773, index #1=0 ("cursor index"), index #2=1 ("cursor index"), index #3=2 ("cursor index")) -> (element #1=w774:i32, element #2=w770:i32, element #3=w768:i32)
        n289 = call "replace cursor - plot ref - V2.vi"("Plot ref in"=w760, "new X"=w767, "cursor index"=w774, "cursor action"=w758, "Color Box"=w757, "cursor state"=w756) -> ("Plot ref out"=w764:refnum<vi>)  [unwired: 10 in, 3 out]
        n290 = call "replace cursor - plot ref - V2.vi"("Plot ref in"=w764, "new X"=w766, "cursor index"=w770, "cursor action"=w758, "Color Box"=w757, "cursor state"=w756) -> ("Plot ref out"=w763:refnum<vi>)  [unwired: 10 in, 3 out]
        n291 = call "replace cursor - plot ref - V2.vi"("Plot ref in"=w763, "new X"=w765, "cursor index"=w768, "cursor action"=w758, "Color Box"=w757, "cursor state"=w756) -> ()  [unwired: 10 in, 4 out]
      }
      frame "color--yellow" {
        w776 = cursor_sate."colored" ("cursor state")
        w777 = u32 16773632 ("Color Box")
        w778 = cursor_action."write"  # action
        n292 = Unbundle By Name(w779) -> ("Plot ref"=w780:refnum<vi>, "cursors"=w793:i32[], "left"=w787:dbl, "center"=w786:dbl, "right"=w785:dbl)
        n293 = Index Array(array=w793, index #1=0 ("cursor index"), index #2=1 ("cursor index"), index #3=2 ("cursor index")) -> (element #1=w794:i32, element #2=w790:i32, element #3=w788:i32)
        n294 = call "replace cursor - plot ref - V2.vi"("Plot ref in"=w780, "new X"=w787, "cursor index"=w794, "cursor action"=w778, "Color Box"=w777, "cursor state"=w776) -> ("Plot ref out"=w784:refnum<vi>)  [unwired: 10 in, 3 out]
        n295 = call "replace cursor - plot ref - V2.vi"("Plot ref in"=w784, "new X"=w786, "cursor index"=w790, "cursor action"=w778, "Color Box"=w777, "cursor state"=w776) -> ("Plot ref out"=w783:refnum<vi>)  [unwired: 10 in, 3 out]
        n296 = call "replace cursor - plot ref - V2.vi"("Plot ref in"=w783, "new X"=w785, "cursor index"=w788, "cursor action"=w778, "Color Box"=w777, "cursor state"=w776) -> ()  [unwired: 10 in, 4 out]
      }
      frame "-write all Y" {
        w812 = cursor_action."write"  # action
        n297 = Unbundle By Name(w800) -> ("Plot ref"=w801:refnum<vi>, "cursors"=w810:i32[])
        n298 = Unbundle By Name(w799) -> ("left.Y"=w798:dbl, "center.Y"=w797:dbl, "right.Y"=w796:dbl)
        n299 = Index Array(array=w810, index #1=0 ("cursor index"), index #2=1 ("cursor index"), index #3=2 ("cursor index")) -> (element #1=w811:i32, element #2=w807:i32, element #3=w805:i32)
        n300 = call "replace cursor - plot ref - V2.vi"("Plot ref in"=w801, "new  Y"=w798, "cursor index"=w811, "cursor action"=w812) -> ("Plot ref out"=w804:refnum<vi>)  [unwired: 12 in, 3 out]
        n301 = call "replace cursor - plot ref - V2.vi"("Plot ref in"=w804, "new  Y"=w797, "cursor index"=w807, "cursor action"=w812) -> ("Plot ref out"=w803:refnum<vi>)  [unwired: 12 in, 3 out]
        n302 = call "replace cursor - plot ref - V2.vi"("Plot ref in"=w803, "new  Y"=w796, "cursor index"=w805, "cursor action"=w812) -> ()  [unwired: 12 in, 4 out]
      }
      frame "-write left.X" {
        w827 = cursor_action."write"  # action
        n303 = Unbundle By Name(w814) -> ("Plot ref"=w819:refnum<vi>, "cursors"=w825:i32[], "left"=w815:dbl, "right"=w816:dbl, "wing order"=w818:enum16{"forw", "back"})
        n304 = Index Array(array=w825, index #1=0 ("cursor index"), index #2=1 ("cursor index"), index #3=2 ("cursor index")) -> (element #1=w826:i32)  [unwired: 2 out]
        n305 = case shown="\"back\"" w818 {
          tunnel: [w829 w830] -> w817
          tunnel: w816 -> [_ w830]
          tunnel: w815 -> [w829 _]
          frame "forw", Default {
          }
          frame "back" {
          }
        }
        n306 = call "replace cursor - plot ref - V2.vi"("Plot ref in"=w819, "new X"=w817, "cursor index"=w826, "cursor action"=w827) -> ()  [unwired: 12 in, 4 out]
      }
      frame "-write right.X" {
        w844 = cursor_action."write"  # action
        n307 = Unbundle By Name(w831) -> ("Plot ref"=w837:refnum<vi>, "cursors"=w843:i32[], "left"=w833:dbl, "right"=w834:dbl, "wing order"=w836:enum16{"forw", "back"})
        n308 = Index Array(array=w843, index #1=0 ("cursor index"), index #2=1 ("cursor index"), index #3=2 ("cursor index")) -> (element #3=w832:i32)  [unwired: 2 out]
        n309 = case shown="\"back\"" w836 {
          tunnel: [w846 w847] -> w835
          tunnel: w834 -> [w846 _]
          tunnel: w833 -> [_ w847]
          frame "forw", Default {
          }
          frame "back" {
          }
        }
        n310 = call "replace cursor - plot ref - V2.vi"("Plot ref in"=w837, "new X"=w835, "cursor index"=w832, "cursor action"=w844) -> ()  [unwired: 12 in, 4 out]
      }
      frame "-write center.X" {
        w858 = cursor_action."write"  # action
        n311 = Unbundle By Name(w850) -> ("Plot ref"=w851:refnum<vi>, "cursors"=w857:i32[], "center"=w848:dbl)
        n312 = Index Array(array=w857, index #1=0 ("cursor index"), index #2=1 ("cursor index"), index #3=2 ("cursor index")) -> (element #2=w849:i32)  [unwired: 2 out]
        n313 = call "replace cursor - plot ref - V2.vi"("Plot ref in"=w851, "new X"=w848, "cursor index"=w849, "cursor action"=w858) -> ()  [unwired: 12 in, 4 out]
      }
      frame "-write center.Y" {
        w870 = cursor_action."write"  # action
        n314 = Unbundle By Name(w863) -> ("Plot ref"=w864:refnum<vi>, "cursors"=w869:i32[])
        n315 = Index Array(array=w869, index #1=0 ("cursor index"), index #2=1 ("cursor index"), index #3=2 ("cursor index")) -> (element #2=w860:i32)  [unwired: 2 out]
        n316 = Unbundle By Name(w862) -> ("center.Y"=w861:dbl)
        n317 = call "replace cursor - plot ref - V2.vi"("Plot ref in"=w864, "new  Y"=w861, "cursor index"=w860, "cursor action"=w870) -> ()  [unwired: 12 in, 4 out]
      }
      frame "-read all cursors" {
        w892 = cursor_action."read"  # action
        n318 = Unbundle By Name(w872) -> ("Plot ref"=w873:refnum<vi>, "cursors"=w890:i32[])
        n319 = Index Array(array=w890, index #1=0 ("cursor index"), index #2=1 ("cursor index"), index #3=2 ("cursor index")) -> (element #1=w891:i32, element #2=w887:i32, element #3=w885:i32)
        n320 = call "replace cursor - plot ref - V2.vi"("Plot ref in"=w873, "cursor index"=w891, "cursor action"=w892) -> ("Plot ref out"=w884:refnum<vi>, "read X"=w880:dbl, "read Y"=w879:dbl)  [unwired: 13 in, 1 out]
        n321 = call "replace cursor - plot ref - V2.vi"("Plot ref in"=w884, "cursor index"=w887, "cursor action"=w892) -> ("Plot ref out"=w883:refnum<vi>, "read X"=w878:dbl, "read Y"=w877:dbl)  [unwired: 13 in, 1 out]
        n322 = call "replace cursor - plot ref - V2.vi"("Plot ref in"=w883, "cursor index"=w885, "cursor action"=w892) -> ("read X"=w876:dbl, "read Y"=w875:dbl)  [unwired: 13 in, 2 out]
        n323 = Bundle By Name(cluster=w882, "left.X"=w880, "left.Y"=w879, "center.X"=w878, "center.Y"=w877, "right.X"=w876, "right.Y"=w875) -> (w881:T3)
      }
      frame "read" {
      }
      frame "-read cursor 2" {
        w910 = cursor_action."read"  # action
        n324 = Unbundle By Name(w899) -> ("Plot ref"=w900:refnum<vi>, "cursors"=w909:i32[])
        n325 = Index Array(array=w909, index #1=0 ("cursor index"), index #2=1 ("cursor index"), index #3=2 ("cursor index")) -> (element #3=w898:i32)  [unwired: 2 out]
        n326 = call "replace cursor - plot ref - V2.vi"("Plot ref in"=w900, "cursor index"=w898, "cursor action"=w910) -> ("read X"=w903:dbl, "read Y"=w902:dbl)  [unwired: 13 in, 2 out]
        n327 = Bundle By Name(cluster=w905, "right.X"=w903, "right.Y"=w902) -> (w904:T3)
      }
      frame "-read cursor 1" {
        w924 = cursor_action."read"  # action
        n328 = Unbundle By Name(w912) -> ("Plot ref"=w914:refnum<vi>, "cursors"=w923:i32[])
        n329 = Index Array(array=w923, index #1=0 ("cursor index"), index #2=1 ("cursor index"), index #3=2 ("cursor index")) -> (element #2=w913:i32)  [unwired: 2 out]
        n330 = call "replace cursor - plot ref - V2.vi"("Plot ref in"=w914, "cursor index"=w913, "cursor action"=w924) -> ("read X"=w917:dbl, "read Y"=w916:dbl)  [unwired: 13 in, 2 out]
        n331 = Bundle By Name(cluster=w919, "center.X"=w917, "center.Y"=w916) -> (w918:T3)
      }
      frame "-read cursor 0" {
        w938 = cursor_action."read"  # action
        n332 = Unbundle By Name(w926) -> ("Plot ref"=w928:refnum<vi>, "cursors"=w937:i32[])
        n333 = Index Array(array=w937, index #1=0 ("cursor index"), index #2=1 ("cursor index"), index #3=2 ("cursor index")) -> (element #1=w927:i32)  [unwired: 2 out]
        n334 = call "replace cursor - plot ref - V2.vi"("Plot ref in"=w928, "cursor index"=w927, "cursor action"=w938) -> ("read X"=w931:dbl, "read Y"=w930:dbl)  [unwired: 13 in, 2 out]
        n335 = Bundle By Name(cluster=w933, "left.X"=w931, "left.Y"=w930) -> (w932:T3)
      }
    }
    n336 = call "cursor window action stack.vi"("stack action"=stack_action_--_control."check", "command stack"=w28) -> ("stack is empty ?"=w26:bool, "command stack out"=w27:T2[])  [unwired: 7 in, 1 out]
  }
  "cursor window out" <- w11
  n337 = property class="Clust (strict)"(reference=w19, "Value"=w11) -> (reference out=→"cursor window out":refnum<vi>)  [unwired: 1 in, 1 out]
